vi "Steuerprogramm-01-17.vi"() -> ()   [LabVIEW 2010]
uses:
  <vilib>/rvi/interface/nirviReadWriteControl/nirviReadWriteControl.xnode
  <vilib>/rvi/errors/niLvFpgaWhatHappensToTopLevelVI.ctl
  <vilib>/rvi/interface/common/niFpgaNodeNameForErrorReporting.ctl
  <vilib>/rvi/errors/niLvFpgaAdjustHostInterfaceError.vi
  gvbooleschRT.vi
  <vilib>/rvi/interface/nirviCloseFPGA/nirviCloseFPGA.xnode
  GVMWHorst.vi
  GVMethodenwechsel.vi
  GVHorstSP.vi
  GVZwangs.vi
  GVHK1Hz.vi
  GVHeizenLH.vi
  GVAIs.vi
  GVTrapsMachs.vi
  GVaktuelleTDMS.vi
  GVECDs.vi
  GVZeitenZyklen.vi
  GVProbenvol.vi
  GVVentilposition.vi
  <vilib>/rvi/interface/nirviMethod/nirviMethod.xnode
  GVChroms.vi
  GVMetavariablen.vi
  GVZwangsMPV.vi
  NiFpgaLv.dll
  <vilib>/Utility/error.llb/Error Cluster From Error Code.vi
  C:/Users/HAGAR-IV/Desktop/Zeugs/markus/version feb 2012/FPGA Bitfiles/pertrasgcfpga2_FPGATarget_FPGA-Programm-01_A75D3647.lvbitx
  C:/Users/HAGAR-IV/Desktop/Zeugs/Johnny/pertrasgc fpga/FPGA-Programm-01-17.vi
  <vilib>/FPGAPlugInAG/cRIO-9114/niLvFpga_Close_cRIO-9114.vi
  Emil/HAGAR V - Licor/control/Licor-Sequences.ctl
  Emil/HAGAR V - Licor/control/Licor-Pump.ctl
  Emil/Licor-Steuerung/LicorLI7000/conventions/Licor-Source.ctl
  Emil/Licor-Steuerung/LicorLI7000/LicorLI7000.lvlib
  Emil/HAGAR V - Licor/control/Licor-Parameter.ctl
panel:
  in  "Methode speichern":bool
  out "ZyklusNummernGesamt":i32[](array[numeric])
  in  "veränderte Methode benutzen":bool
  in  "Methode verändern":bool
  out "ZyklusNummern":i32[](array[numeric])
  out "Big Ben, Methodenzeit, Zykluszeit0, Zykluszeit1, Zykluszeit2A, Zykluszeit2B":i32[](array[numeric])
  in  "global stop RT":bool
  in  "Methode":i32(ring) items=["Bedingsmethode", "Startmethode", "Meßmodus", "Shut-up-Methode", "Test", "HAG2 1/2", "Startmethode", "HAG2 1/2 Aufwärmen"]
  in  "Registerkarte":T1(tab)
  out "AIs1":dbl[](array[numeric])
  out "AIs1":string[](array[string])
  out "AIs2":string[](array[string])
  out "AIs3":string[](array[string])
  out "AIs2":dbl[](array[numeric])
  out "AIs3":dbl[](array[numeric])
  out "Metavariablen":string[](array[string])
  out "Metavariablen":dbl[](array[numeric])
  out "MWHorst":dbl[](array[numeric])
  out "HorstRegler":string[](array[string])
  out "Ventilposition":i32=1 min=1 max=6 step=1
  out "Housekeeping1":cluster{dbl[], dbl[]}(graph)
  in  "Zeitachse1":i32(ring)=1 items=["Zykluszeit [s] Mod0", "Zykluszeit [s] Mod1", "Zykluszeit [s] Mod2A", "Zykluszeit [s] Mod2B"]
  in  "dargestellte Größe 1":i32(ring)=1 items=["T1-Trap1", "T1-Trap2", "T1-StirlingKühlkopf", "T1-PreCol1", "T1-PreCol2", "T1-MainCol1a", "T1-MainCol1b", "T1-MainCol2a", "T1-MainCol2b", "T1-Bronkhorst1a", "T1-Bronkhorst1b", "T1-Bronkhorst2a", "T1-Bronkhorst2b", "T1-2Pos1B", "T1-Spare9", "T1-2Pos1A", "T1-Spare10", "T1-TurboPump", "T1-StirlingPlatine", "T1-Spare5", "T1-Spare6", "T1-Spare7", "T1-Spare8", "F1-MFM1", "F1-MFM0D [mL]", "P1-MethaneHP", "P1-MethaneLP", "P1-Vacuum", "TurboSpeed", "I1-MS-AC", "I1-Trap1", "I1-Trap2", "T2-ECD1a", "T2-ECD1b", "T2-ECD2a", "T2-ECD2b", "T2-Col1a", "T2-Col1b", "T2-Col2a", "T2-Col2b", "T2-Spare1", "T2-Spare2", "T2-Oven_a", "T2-Oven_b", "T2-Spare3", "T2-Spare4", "T2-Spare5", "F2-MFM0", "F2-MFM2A", "F2-MFM2B", "P2-N2O_HP", "P2-N2O_LP", "P2-CO2_HP", "P2-CO2_LP", "AI-Spare1", "FL-MFM1000mL", "AI-Spare3", "AI-Spare4", "StirlingAlarm", "StirlingEmerg.", "AI-Spare7", "AI-Spare8", "AI-Spare9", "FL-MFM30mL", "T0-DC/DC5", "I0-24V_M0", "I0-48V_M1", "I0-24V_M1", "I0-28V_M2", "T0-Spare3", "T0-Spare2", "T0-Spare4", "T0-DC/DC7", "I0-20V_Laptop", "I0-28V_M1", "I0-24V_M2", "I0-12V_Licor", "T0-Spare1", "T0-Drier", "T0-Spare5", "F0-MFM0A [L]", "TL-Licor_a", "P0-Span-HP", "P0-spare1", "P0-Stickstoff-LP", "P0-Helium-LP", "P0-Cal-HP", "P0-P9Tavco[bar]", "F0-MFM0B [L]", "TL-Licor_b", "P0-Span-LP", "P0-spare2", "P0-Stickstoff-HP", "P0-Helium-HP", "P0-Cal-LP", "F0-MFM3", "TemperaturTrap1[°C]", "TemperaturTrap2[°C]", "TemperaturPreMach1[°C]", "TemperaturPreMach2[°C]", "TemperaturMainMach1[°C]", "TemperaturMainMach2[°C]", "PrC0", "PrC0-Licor", "PrC1-Säule2", "PrC1-Säule1", "MFC1-Sample", "MFC1-Methan", "PrC1-BackFlush1", "PrC1-BackFlush2", "MFC2A", "MFC2B", "MFC2C", "PrC2A", "MFC2D", "MFC2E", "PrC2B"]
  out "Housekeeping2":cluster{dbl[], dbl[]}(graph)
  in  "Zeitachse2":i32(ring)=1 items=["Zykluszeit [s] Mod0", "Zykluszeit [s] Mod1", "Zykluszeit [s] Mod2A", "Zykluszeit [s] Mod2B"]
  in  "dargestellte Größe 2":i32(ring)=1 items=["T1-Trap1", "T1-Trap2", "T1-StirlingKühlkopf", "T1-PreCol1", "T1-PreCol2", "T1-MainCol1a", "T1-MainCol1b", "T1-MainCol2a", "T1-MainCol2b", "T1-Bronkhorst1a", "T1-Bronkhorst1b", "T1-Bronkhorst2a", "T1-Bronkhorst2b", "T1-2Pos1B", "T1-Spare9", "T1-2Pos1A", "T1-Spare10", "T1-TurboPump", "T1-StirlingPlatine", "T1-Spare5", "T1-Spare6", "T1-Spare7", "T1-Spare8", "F1-MFM1", "F1-MFM0D [mL]", "P1-MethaneHP", "P1-MethaneLP", "P1-Vacuum", "TurboSpeed", "I1-MS-AC", "I1-Trap1", "I1-Trap2", "T2-ECD1a", "T2-ECD1b", "T2-ECD2a", "T2-ECD2b", "T2-Col1a", "T2-Col1b", "T2-Col2a", "T2-Col2b", "T2-Spare1", "T2-Spare2", "T2-Oven_a", "T2-Oven_b", "T2-Spare3", "T2-Spare4", "T2-Spare5", "F2-MFM0", "F2-MFM2A", "F2-MFM2B", "P2-N2O_HP", "P2-N2O_LP", "P2-CO2_HP", "P2-CO2_LP", "AI-Spare1", "FL-MFM1000mL", "AI-Spare3", "AI-Spare4", "StirlingAlarm", "StirlingEmerg.", "AI-Spare7", "AI-Spare8", "AI-Spare9", "FL-MFM30mL", "T0-DC/DC5", "I0-24V_M0", "I0-48V_M1", "I0-24V_M1", "I0-28V_M2", "T0-Spare3", "T0-Spare2", "T0-Spare4", "T0-DC/DC7", "I0-20V_Laptop", "I0-28V_M1", "I0-24V_M2", "I0-12V_Licor", "T0-Spare1", "T0-Drier", "T0-Spare5", "F0-MFM0A [L]", "TL-Licor_a", "P0-Span-HP", "P0-spare1", "P0-Stickstoff-LP", "P0-Helium-LP", "P0-Cal-HP", "P0-P9Tavco[bar]", "F0-MFM0B [L]", "TL-Licor_b", "P0-Span-LP", "P0-spare2", "P0-Stickstoff-HP", "P0-Helium-HP", "P0-Cal-LP", "F0-MFM3", "TemperaturTrap1[°C]", "TemperaturTrap2[°C]", "TemperaturPreMach1[°C]", "TemperaturPreMach2[°C]", "TemperaturMainMach1[°C]", "TemperaturMainMach2[°C]", "PrC0", "PrC0-Licor", "PrC1-Säule2", "PrC1-Säule1", "MFC1-Sample", "MFC1-Methan", "PrC1-BackFlush1", "PrC1-BackFlush2", "MFC2A", "MFC2B", "MFC2C", "PrC2A", "MFC2D", "MFC2E", "PrC2B"]
  out "Detektor 2":cluster{dbl[], dbl[]}[](graph)
  in  "Detektor":i32(ring) items=["ECD1", "ECD2"]
  in  "HK1YMin":dbl
  in  "HK1YMax":dbl=100.0
  in  "HK2YMin":dbl
  in  "HK2YMax":dbl=100.0
  in  "DetYMin":dbl
  in  "DetYMax":dbl=100.0
  out "schnelleAnzeige":cluster{dbl[], dbl[]}(graph)
  in  "TafelWischen!":bool
  in  "dargestellte Größe 3":i32(ring)=1 items=["TemperaturTrap1[°C]", "TemperaturTrap2[°C]", "TemperaturPreMach1[°C]", "TemperaturPreMach2[°C]", "TemperaturMainMach1[°C]", "TemperaturMainMach2[°C]", "PrC0", "PrC0-Licor", "PrC1-Säule2", "PrC1-Säule1", "MFC1-Sample", "MFC1-Methan", "PrC1-BackFlush1", "PrC1-BackFlush2", "MFC2A", "MFC2B", "MFC2C", "PrC2A", "MFC2D", "MFC2E", "PrC2B"]
  in  "An/Aus":bool
  in  "manual control":T3={"sequence manual"=enum."WAIT", "sequence manual ?"=FALSE}
  out "Licor-output":string[](array[string])
  out "graph":cluster{"X":dbl[], "Y":dbl[]}(graph)
  in  "Licor-parameter out":T4={"CO2 ref"=392.0, "CO2 span"=402.0, "H2O ref"=0.0, "H2O span"=0.0, "Zi"=1.2, "Zt"=0.0, "Zm"=0.0, "S"=1.0, "Temp [C]"=50.0, "Pressure [hPa]"=135.0, "Licor-Sources"=["CO2A W", "CO2B W", "H2OA W", "H2OB W", "T C", "T V", "P kPa", "P V", "RH %", "CO2A um/m", "CO2B um/m", "H2OA mm/m", "H2OB mm/m"], "Licor-Pump"="Off", "Zeitstempel"=timestamp(0 s since 1904-01-01)} {"Pressure [hPa]" format="%.2g"; "Temp [C]" format="%.2f"; "CO2 ref" format="%.2f"; "CO2 span" format="%.2g"; "H2O ref" format="%.2g"; "H2O span" format="%.2g"}
  in  "ServosWarmHigh (us)KaltHigh(us)":T7={"Servo1WarmHigh(us)"=1000, "Servo1KaltHigh(us)"=1000, "Servo2WarmHigh(us)"=2030, "Servo2KaltHigh(us)"=2030}
  out "TDMSwriteECD":errorcluster
  out "AIsFIFOread":errorcluster
  out "MWTrapsMachs":errorcluster
  out "TDMSwriteHK":errorcluster
  out "TDMScloseHK":errorcluster
  out "TDMSopenHK":errorcluster
  out "TDMScloseECD2":errorcluster
  out "TDMSopenECD2":errorcluster
  out "TDMScloseECD1":errorcluster
  out "TDMSopenECD1":errorcluster
  out "FIFOwriteRS485":errorcluster
  out "SerielleKomm.":errorcluster
  out "LH":errorcluster
  out "Zyklus":errorcluster
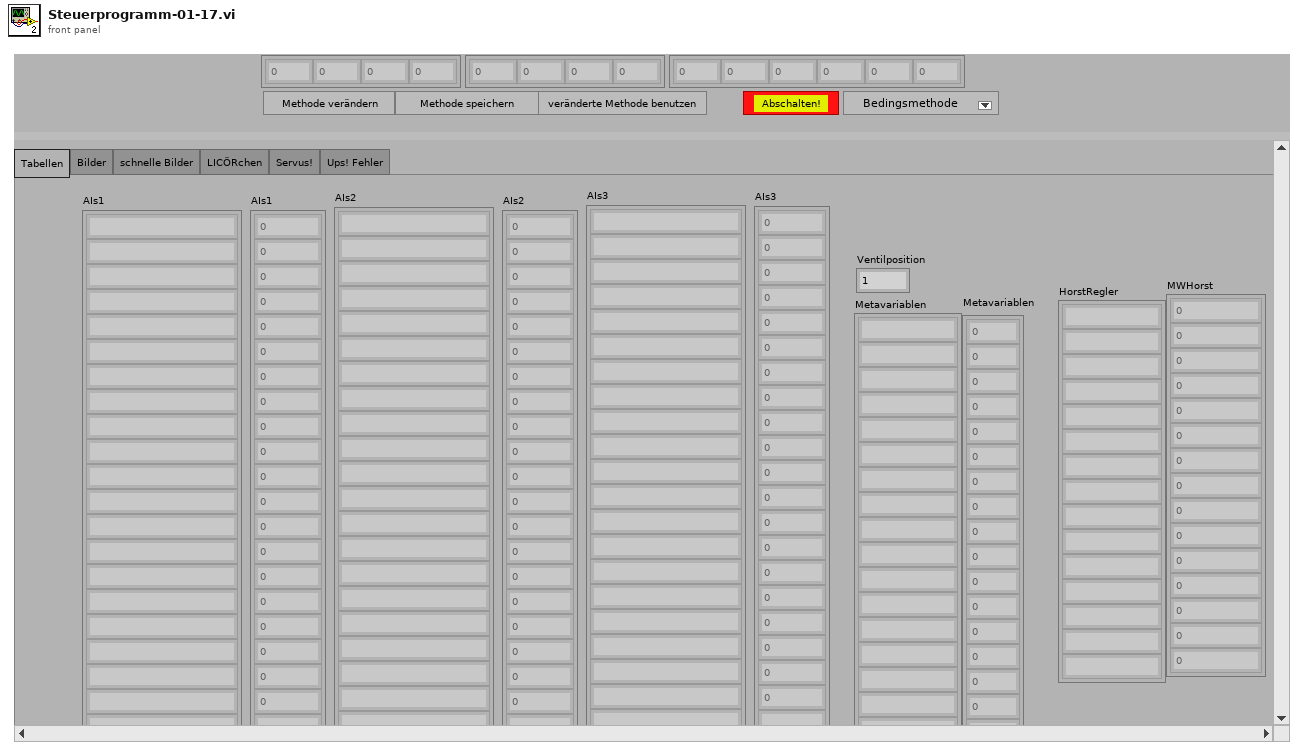
[diagram p1: front panel]
types:
  T1 = enum32{"Tabellen", "Bilder", "schnelle Bilder", "LICÖRchen", "Servus!", "Ups! Fehler"}
  T2 = typedef "Licor-Sequences.ctl" = enum16{"test", "WAIT", "warmup", "initialize", "calibrate Z", "calibrate S"}
  T3 = cluster{"sequence manual":T2, "sequence manual ?":bool}
  T4 = typedef "Licor-Parameter.ctl" = cluster{"CO2 ref":dbl, "CO2 span":dbl, "H2O ref":dbl, "H2O span":dbl, "Zi":dbl, "Zt":dbl, "Zm":dbl, "S":dbl, "Temp [C]":dbl, "Pressure [hPa]":dbl, "Licor-Sources":T5[], "Licor-Pump":T6, "Zeitstempel":timestamp}
  T5 = typedef "LicorLI7000.lvlib/Licor-Source.ctl" = string
  T6 = typedef "Licor-Pump.ctl" = string
  T7 = cluster{"Servo1WarmHigh(us)":u32, "Servo1KaltHigh(us)":u32, "Servo2WarmHigh(us)":u32, "Servo2KaltHigh(us)":u32}
  T8 = cluster{"DIOsMod0Nr":i32[], "DIOsMod1Nr":i32[], "DIOsMod2ANr":i32[], "DIOsMod2BNr":i32[], "AIsLH":i32[], "AnzahlRegler/Modul":i32[], "Regler für den Probenfluß":i32, "SPvorgebenMod0":string[], "SPvorgebenMod1":string[], "SPvorgebenMod2A":string[], "SPvorgebenMod2B":string[], "MWAntwortMod0":string[], "MWAntwortMod1":string[], "MWAntwortMod2A":string[], "MWAntwortMod2B":string[], "FaktorMod0":dbl[], "FaktorMod1":dbl[], "FaktorMod2A":dbl[], "FaktorMod2B":dbl[], "MWabfragenMod0":string[], "MWabfragenMod1":string[], "MWabfragenMod2A":string[], "MWabfragenMod2B":string[], "Modul1/AI koeff":dbl[][], "Modul2/AI koeff":dbl[][], "Modul3/AI koeff":dbl[][], "Traps/MachsKoeff":dbl[][], "Modul1/AIsNamen":string[], "Modul2/AIsNamen":string[], "Modul3/AIsNamen":string[], "DIOsMod0Name":string[], "DIOsMod1Name":string[], "DIOsMod2AName":string[], "DIOsMod2BName":string[], "ReglerNameMod0":string[], "ReglerNameMod1":string[], "ReglerNameMod2A":string[], "ReglerNameMod2B":string[], "Startmethode":i32, "Dateiordner Housekeeping":path, "Dateiname Housekeeping":string, "DateiordnerECD1":path, "DateinameECD1":string, "DateiordnerECD2":path, "DateinameECD2":string, "NamenLangsameHeizungen":string[], "ModuleLH":i32[], "Metavariablen":string[]}
  T9 = cluster{"Zykluslängen [s]":dbl[], "ZeitpktDIOsMod0":dbl[], "ZeitpktDIOsMod1":dbl[], "ZeitpktDIOsMod2A":dbl[], "ZeitpktDIOsMod2B":dbl[], "DIOsSPMod0":bool[][], "DIOsSPMod1":bool[][], "DIOsSPMod2A":bool[][], "DIOsSPMod2B":bool[][], "Mod0HorstZeitpkt":dbl[], "Mod1HorstZeitpkt":dbl[], "Mod2AHorstZeitpkt":dbl[], "Mod2BHorstZeitpkt":dbl[], "HorstSPMod0":dbl[][], "HorstSPMod1":dbl[][], "HorstSPMod2A":dbl[][], "HorstSPMod2B":dbl[][], "LHSetpoints":dbl[], "LHHeizen?":bool[], "ZPktFPGABoolesch":dbl[], "FPGABoolesch":bool[][], "ZeitpktFPGAPID":dbl[], "FPGAPID":cluster{"proportional gain (Kc)":fxp<+/-,16,8>, "integral gain (Kc*Ts/Ti)":fxp<+/-,16,8>, "derivative gain (Kc*Td/Ts)":fxp<+/-,16,8>}[][], "ZeitpktFPGAFixp":dbl[], "SHSetpoints":dbl[][], "t_PreMach1":dbl[], "T_PreMach1":dbl[], "t_PreMach2":dbl[], "T_PreMach2":dbl[], "PIDs für \"träge\" Heizungen":cluster{"proportional gain (Kc)":dbl, "integral time (Ti, min)":dbl, "derivative time (Td, min)":dbl}[], "Zwangsbedingungen":dbl[][], "Dateien fürs MS schicken?":bool, "ZeitpunkteMPV":dbl[], "SPMPV":i32[], "ZeitpktMS-1":dbl, "ZeitpktMS-2":dbl, "Int.Start1":dbl, "Int.Stop1":dbl, "Int.Start2":dbl, "Int.Stop2":dbl, "Methodenname":string, "t_MainMach1":dbl[], "T_MainMach1":dbl[], "t_MainMach2":dbl[], "T_MainMach2":dbl[]}[]
  T10 = enum16{"open", "replace", "create", "open or create", "replace or create", "replace or create with confirmation"}
  T11 = typedef "niFpgaNodeNameForErrorReporting.ctl" = enum16{"Open FPGA VI Reference", "Read/Write Control", "Invoke Method: Abort", "Invoke Method: Acknowledge IRQ", "Invoke Method: Download", "Invoke Method: FIFO.Configure", "Invoke Method: FIFO.Read", "Invoke Method: FIFO.Start", "Invoke Method: FIFO.Stop", "Invoke Method: FIFO.Write", "Invoke Method: Reset", "Invoke Method: Run", "Invoke Method: Wait on IRQ", "Close FPGA VI Reference"}
  T12 = typedef "niLvFpgaWhatHappensToTopLevelVI.ctl" = enum16{"top level VI scripted behind XNode", "top level VI inlined behind XNode"}
  T13 = cluster{"Zyklus1":i32, "Zeitachse1":i32, "dargestellte Größe 1":i32, "Zyklus2":i32, "Zeitachse2":i32, "dargestellte Größe 2":i32}
  T14 = cluster{"DIOsMod0Name":string[], "DIOsMod1Name":string[], "DIOsMod2AName":string[], "DIOsMod2BName":string[], "ReglerNameMod0":string[], "ReglerNameMod1":string[], "ReglerNameMod2A":string[], "ReglerNameMod2B":string[], "NamenLangsameHeizungen":string[]}
  T15 = cluster{"Zykluslängen [s]":dbl[], "ZeitpktDIOsMod0":dbl[], "ZeitpktDIOsMod1":dbl[], "ZeitpktDIOsMod2A":dbl[], "ZeitpktDIOsMod2B":dbl[], "DIOsSPMod0":bool[][], "DIOsSPMod1":bool[][], "DIOsSPMod2A":bool[][], "DIOsSPMod2B":bool[][], "Mod0HorstZeitpkt":dbl[], "Mod1HorstZeitpkt":dbl[], "Mod2AHorstZeitpkt":dbl[], "Mod2BHorstZeitpkt":dbl[], "HorstSPMod0":dbl[][], "HorstSPMod1":dbl[][], "HorstSPMod2A":dbl[][], "HorstSPMod2B":dbl[][], "LHSetpoints":dbl[], "LHHeizen?":bool[], "ZPktFPGABoolesch":dbl[], "FPGABoolesch":bool[][], "ZeitpktFPGAPID":dbl[], "FPGAPID":cluster{"proportional gain (Kc)":fxp<+/-,16,8>, "integral gain (Kc*Ts/Ti)":fxp<+/-,16,8>, "derivative gain (Kc*Td/Ts)":fxp<+/-,16,8>}[][], "ZeitpktFPGAFixp":dbl[], "SHSetpoints":dbl[][], "t_PreMach1":dbl[], "T_PreMach1":dbl[], "t_PreMach2":dbl[], "T_PreMach2":dbl[], "PIDs für \"träge\" Heizungen":cluster{"proportional gain (Kc)":dbl, "integral time (Ti, min)":dbl, "derivative time (Td, min)":dbl}[], "Zwangsbedingungen":dbl[][], "Dateien fürs MS schicken?":bool, "ZeitpunkteMPV":dbl[], "SPMPV":i32[], "ZeitpktMS-1":dbl, "ZeitpktMS-2":dbl, "Int.Start1":dbl, "Int.Stop1":dbl, "Int.Start2":dbl, "Int.Stop2":dbl, "Methodenname":string, "t_MainMach1":dbl[], "T_MainMach1":dbl[], "t_MainMach2":dbl[], "T_MainMach2":dbl[]}
  T16 = cluster{"created path":path, "created path":path, "created path":path, "Dateiname Housekeeping":string, "DateinameECD1":string, "DateinameECD2":string, "tdms0":refnum<k34>, "tdms1":refnum<k34>, "tdms0":refnum<k34>, "tdms1":refnum<k34>, "tdms0":refnum<k34>, "tdms1":refnum<k34>}
  T17 = cluster{"proportional gain (Kc)":fxp<+/-,16,8>, "integral gain (Kc*Ts/Ti)":fxp<+/-,16,8>, "derivative gain (Kc*Td/Ts)":fxp<+/-,16,8>}[][]
  T18 = cluster{"proportional gain (Kc)":dbl, "integral time (Ti, min)":dbl, "derivative time (Td, min)":dbl}[]
  T19 = cluster{cluster{"ZeitpktDIOsMod2B":dbl[]}[], cluster{"DIOsSPMod2B":bool[][]}[], cluster{"Mod2BHorstZeitpkt":dbl[]}[], cluster{"HorstSPMod2B":dbl[][]}[], "LHHeizen?":bool[], "ZPktFPGABoolesch":dbl[], "FPGABoolesch":bool[][], "ZeitpktFPGAPID":dbl[], "FPGAPID":cluster{"proportional gain (Kc)":fxp<+/-,16,8>, "integral gain (Kc*Ts/Ti)":fxp<+/-,16,8>, "derivative gain (Kc*Td/Ts)":fxp<+/-,16,8>}[][], "ZeitpktFPGAFixp":dbl[], "SHSetpoints":dbl[][], "t_PreMach1":dbl[], "T_PreMach1":dbl[], "t_PreMach2":dbl[], "T_PreMach2":dbl[], "ZeitpunkteMPV":dbl[], "SPMPV":i32[], "t_MainMach1":dbl[], "T_MainMach1":dbl[], "t_MainMach2":dbl[], "T_MainMach2":dbl[]}
  T20 = cluster{"Zykluslängen [s]":dbl[], "ZeitpktDIOsMod0":dbl[], "ZeitpktDIOsMod1":dbl[], "ZeitpktDIOsMod2A":dbl[], "ZeitpktDIOsMod2B":dbl[], "DIOsSPMod0":bool[][], "DIOsSPMod1":bool[][], "DIOsSPMod2A":bool[][], "DIOsSPMod2B":bool[][], "Mod0HorstZeitpkt":dbl[], "Mod1HorstZeitpkt":dbl[], "Mod2AHorstZeitpkt":dbl[], "Mod2BHorstZeitpkt":dbl[], "HorstSPMod0":dbl[][], "HorstSPMod1":dbl[][], "HorstSPMod2A":dbl[][], "HorstSPMod2B":dbl[][], "LangsameHeizungenSP":dbl[], "LHHeizen?":bool[], "ZPktFPGABoolesch":dbl[], "FPGABoolesch":bool[][], "ZeitpktFPGAPID":dbl[], "FPGAPID":cluster{"proportional gain (Kc)":fxp<+/-,16,8>, "integral gain (Kc*Ts/Ti)":fxp<+/-,16,8>, "derivative gain (Kc*Td/Ts)":fxp<+/-,16,8>}[][], "ZeitpktFPGAFixp":dbl[], "FPGAFixp":dbl[][], "t_PreMach1":dbl[], "T_PreMach1":dbl[], "t_PreMach2":dbl[], "T_PreMach2":dbl[], "PIDs für \"träge\" Heizungen":cluster{"proportional gain (Kc)":dbl, "integral time (Ti, min)":dbl, "derivative time (Td, min)":dbl}[], "Zwangsbedingungen":dbl[][], "MS-Daten?":bool, "ZeitpunkteMPV":dbl[], "SetpointMPV":i32[], "ZeitpktMS-1":dbl, "ZeitpktMS-2":dbl, "Int.Start1":dbl, "Int.Stop1":dbl, "Int.Start2":dbl, "Int.Stop2":dbl, "Methodenname":string, "t_MainMach1":dbl[], "T_MainMach1":dbl[], "t_MainMach2":dbl[], "T_MainMach2":dbl[]}
  T21 = cluster{"ZyklusNummern":i32[], "ZeilennummernDIOs":i32[], "ZwangsDIO?":cluster{bool[]}[], "ZeilennummernHorst":i32[], "ZwangsHorst?":cluster{bool[]}[], "ZeileFPGABoolesch":i32, "ZwangsFPGABoolesch?":bool[], "ZeileFPGAPID":i32, "ZeileFPGAFixp":i32, "ZeilePreMach1":i32, "ZeilePreMach2":i32, "ZeilennummerMPV":i32, "ZeileMainMach1":i32, "ZeileMainMach2":i32, "ZwangsMPV?":bool}
  T22 = cluster{"ZyklusNummern":i32[], i32[], "ZwangsDIO?":cluster{bool[]}[], i32[], "ZwangsHorst?":cluster{bool[]}[], i32, "ZwangsFPGABoolesch?":bool[], i32, i32, "ZeileMach":i32, "ZeileMach":i32, i32, "ZeileMach":i32, "ZeileMach":i32, "ZwangsMPV?":bool}
  T23 = cluster{string[], string[], string[], dbl[], dbl[], dbl[]}
  T24 = cluster{"Befehle1":string[], "Befehle2":string[], "Befehle3":string[]}
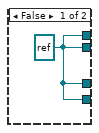
[diagram p2: hidden frame]
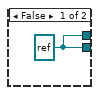
[diagram p3: hidden frame]
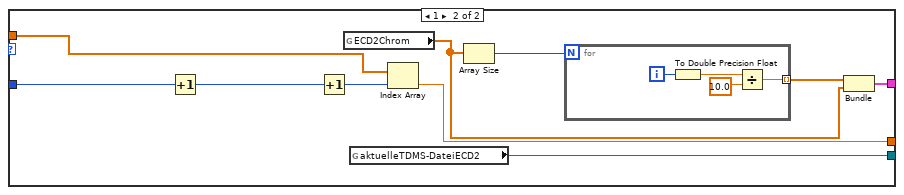
[diagram p13: hidden frame]
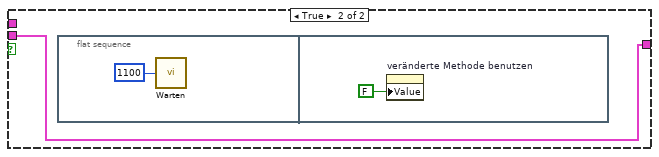
[diagram p14: hidden frame]
diagram:
  n1 = Open/Create/Replace File(file path (use dialog)=path "c:/einstellungen.per" ("Datei (Dialog verwenden)"), operation (0:open)=T10."open" ("Operation (0:Öffnen)")) -> (refnum out=w12:refnum<file>)  [unwired: 4 in, 2 out]
  n2 = Open/Create/Replace File(file path (use dialog)=path "c:/methoden.per" ("Datei (Dialog verwenden)"), operation (0:open)=T10."open" ("Operation (0:Öffnen)")) -> (refnum out=w7:refnum<file>)  [unwired: 4 in, 2 out]
  n3 = Read from Binary File(5:T8 {"DIOsMod0Nr"=[], "DIOsMod1Nr"=[], "DIOsMod2ANr"=[], "DIOsMod2BNr"=[], "AIsLH"=[], "AnzahlRegler/Modul"=[], "Regler für den Probenfluß"=0, "SPvorgebenMod0"=[], "SPvorgebenMod1"=[], "SPvorgebenMod2A"=[], "SPvorgebenMod2B"=[], "MWAntwortMod0"=[], "MWAntwortMod1"=[], "MWAntwortMod2A"=[], "MWAntwortMod2B"=[], "FaktorMod0"=[], "FaktorMod1"=[], "FaktorMod2A"=[], "FaktorMod2B"=[], "MWabfragenMod0"=[], "MWabfragenMod1"=[], "MWabfragenMod2A"=[], "MWabfragenMod2B"=[], "Modul1/AI koeff"=[], "Modul2/AI koeff"=[], "Modul3/AI koeff"=[], "Traps/MachsKoeff"=[], "Modul1/AIsNamen"=[], "Modul2/AIsNamen"=[], "Modul3/AIsNamen"=[], "DIOsMod0Name"=[], "DIOsMod1Name"=[], "DIOsMod2AName"=[], "DIOsMod2BName"=[], "ReglerNameMod0"=[], "ReglerNameMod1"=[], "ReglerNameMod2A"=[], "ReglerNameMod2B"=[], "Startmethode"=0, "Dateiordner Housekeeping"=path "", "Dateiname Housekeeping"="", "DateiordnerECD1"=path "", "DateinameECD1"="", "DateiordnerECD2"=path "", "DateinameECD2"="", "NamenLangsameHeizungen"=[], "ModuleLH"=[], "Metavariablen"=[]} ("Ausgangs-Cluster"), 11:w12) -> (2:w10:T8, 3:w11:refnum<file>)  [unwired: 4 in, 2 out]
  n4 = Read from Binary File(5:T9 [], 11:w7) -> (2:w5:T9, 3:w6:refnum<file>)  [unwired: 4 in, 2 out]
  n5 = Close File(refnum=w11) -> ()  [unwired: 1 in, 2 out]
  n6 = Close File(refnum=w6) -> ()  [unwired: 1 in, 2 out]
  n7 = flat-sequence {
    tunnel: [w41] -> w40
    tunnel: [w98] -> w39
    tunnel: [w45] -> w37
    tunnel: [w232] -> w36
    tunnel: [w234] -> w35
    tunnel: [w226] -> w34
    tunnel: [w233] -> w33
    tunnel: [w156] -> w32
    tunnel: [w225] -> w31
    tunnel: [w224] -> w30
    tunnel: [w218] -> w29
    tunnel: [w159] -> w28
    tunnel: [w133] -> w27
    tunnel: [w231] -> w26
    tunnel: [w223] -> w25
    tunnel: [w222] -> w24
    tunnel: [w214] -> w23
    tunnel: [w213] -> w22
    tunnel: [w212] -> w21
    tunnel: [w211] -> w20
    tunnel: [w210] -> w19
    tunnel: [w209] -> w18
    tunnel: [w206] -> w17
    tunnel: [w188] -> w16
    tunnel: w10 -> [w74]
    tunnel: [w187] -> w15
    tunnel: w5 -> [w99]
    tunnel: [w98] -> w4
    tunnel: [w74] -> w1
    tunnel: w40 -> [w430]
    tunnel: w39 -> [w503]
    tunnel: [w430] -> w38
    tunnel: w37 -> [_]
    tunnel: w36 -> [w461]
    tunnel: w35 -> [w460]
    tunnel: w34 -> [w462]
    tunnel: w33 -> [w459]
    tunnel: w32 -> [w434]
    tunnel: w31 -> [w429]
    tunnel: w30 -> [w426]
    tunnel: w29 -> [w423]
    tunnel: w28 -> [w424]
    tunnel: w27 -> [w427]
    tunnel: w26 -> [w501]
    tunnel: w25 -> [w432]
    tunnel: w24 -> [w502]
    tunnel: w23 -> [w405]
    tunnel: w22 -> [w404]
    tunnel: w21 -> [w403]
    tunnel: w20 -> [w499]
    tunnel: w19 -> [w498]
    tunnel: w18 -> [w497]
    tunnel: w17 -> [w451]
    tunnel: w16 -> [w433]
    tunnel: w15 -> [w422]
    tunnel: w5 -> [w421]
    tunnel: w4 -> [w419]
    tunnel: w1 -> [_]
    tunnel: w38 -> [w1270]
    frame #0 {
      w100 = TRUE
      w115 = 0.0 ("Probenvol.1")
      w122 = dbl[] [-1.0] ("ECD1MW")
      w123 = FALSE ("ECD1Empfangen?")
      w114 = string[] ["TemperaturTrap1[°C]", "TemperaturTrap2[°C]", "TemperaturPreMach1[°C]", "TemperaturPreMach2[°C]", "TemperaturMainMach1[°C]", "TemperaturMainMach2[°C]"]
      w229 = string[] ["Big Ben [s]", "Methodenzeit [s]", "Zykluszeit [s] Mod0", "Zykluszeit [s] Mod1", "Zykluszeit [s] Mod2A", "Zykluszeit [s] Mod2B"]
      w219 = FALSE ("Undefinierte Werte möglich")
      w220 = FALSE ("global stop RT")
      n8 = for {
        tunnel: [w394] -> w227 mode=indexing
        tunnel: w99 -> [w395] mode=indexing
        n9 = Unbundle(w395) -> ("Methodenname"=w394:string)  [unwired: 44 out]
      }
      n10 = call "FPGA-Start-01-17.vi"() -> ("error out"=w45:errorcluster, "FPGA VI Reference Out"=w44:refnum<k20>)  [unwired: 2 in]
      n11 = Unbundle(w74) -> ("DIOsMod0Nr"=w143:i32[], "DIOsMod1Nr"=w142:i32[], "DIOsMod2ANr"=w141:i32[], "DIOsMod2BNr"=w140:i32[], "AIsLH"=w130:i32[], "AnzahlRegler/Modul"=w133:i32[], "Regler für den Probenfluß"=w187:i32, "SPvorgebenMod0"=w186:string[], "SPvorgebenMod1"=w185:string[], "SPvorgebenMod2A"=w184:string[], "SPvorgebenMod2B"=w183:string[], "MWAntwortMod0"=w182:string[], "MWAntwortMod1"=w181:string[], "MWAntwortMod2A"=w180:string[], "MWAntwortMod2B"=w179:string[], "FaktorMod0"=w178:dbl[], "FaktorMod1"=w177:dbl[], "FaktorMod2A"=w176:dbl[], "FaktorMod2B"=w175:dbl[], "MWabfragenMod0"=w174:string[], "MWabfragenMod1"=w173:string[], "MWabfragenMod2A"=w172:string[], "MWabfragenMod2B"=w171:string[], "Modul1/AI koeff"=w170:dbl[][], "Modul2/AI koeff"=w169:dbl[][], "Modul3/AI koeff"=w168:dbl[][], "Traps/MachsKoeff"=w167:dbl[][], "Modul1/AIsNamen"=w166:string[], "Modul2/AIsNamen"=w165:string[], "Modul3/AIsNamen"=w164:string[], "DIOsMod0Name"=w72:string[], "DIOsMod1Name"=w73:string[], "DIOsMod2AName"=w71:string[], "DIOsMod2BName"=w70:string[], "ReglerNameMod0"=w89:string[], "ReglerNameMod1"=w88:string[], "ReglerNameMod2A"=w87:string[], "ReglerNameMod2B"=w86:string[], "Startmethode"=w98:i32, "Dateiordner Housekeeping"=w69:path, "Dateiname Housekeeping"=w163:string, "DateiordnerECD1"=w83:path, "DateinameECD1"=w162:string, "DateiordnerECD2"=w82:path, "DateinameECD2"=w161:string, "NamenLangsameHeizungen"=w160:string[], "ModuleLH"=w155:i32[], "Metavariablen"=w93:string[])
      "Metavariablen" <- w93
      n12 = Initialize Array(0, 4 ("Dimension")) -> (w116:i32[])
      n13 = Initialize Array(0.0 ("Element"), 6 ("Dimension")) -> (w119:dbl[])
      n14 = global write "GVMethodenwechsel.vi" "Methodenwechsel?"(FALSE ("Methodenwechsel?")) -> ()
      n15 = Concatenate Strings("?SE0,SETP,2200" ("string"), "\r\n") -> (w47:string)
      n16 = Concatenate Strings("?SE0,SETP,2300" ("string"), "\r\n") -> (w54:string)
      n17 = String To Byte Array(string=w54) -> (unsigned byte array=w59:u8[])
      n18 = Join Numbers(hi=w59, lo=u8 6) -> ((hi.lo)=w57:u16[])
      n19 = String To Byte Array(string=w47) -> (unsigned byte array=w49:u8[])
      n20 = Join Numbers(hi=w49, lo=u8 5) -> ((hi.lo)=w46:u16[])
      n21 = xnode "Invoke Method"("FPGA VI Reference In"=w44, "Data"=w46) -> ("FPGA VI Reference Out"=w52:refnum<k20>)  [unwired: 2 in, 2 out]
      n22 = xnode "Invoke Method"("FPGA VI Reference In"=w52, "Data"=w57) -> ("FPGA VI Reference Out"=w43:refnum<k20>)  [unwired: 2 in, 2 out]
      n23 = global write "GVProbenvol.vi" "Probenvol.1"(w115) -> ()
      n24 = global write "GVProbenvol.vi" "Probenvol.2"(w115) -> ()
      n25 = global write "GVECDs.vi" "ECD1MW"(w122) -> ()
      n26 = global write "GVECDs.vi" "ECD2MW"(w122) -> ()
      n27 = global write "GVECDs.vi" "ECD1Empfangen?"(w123) -> ()
      n28 = global write "GVECDs.vi" "ECD2Empfangen?"(w123) -> ()
      n29 = property on="dargestellte Größe 2" class="Ring (strict)"("AllowUndefVals"=w219) -> ()  [unwired: 2 in, 2 out]
      n30 = property on="Zeitachse2" class="Ring (strict)"("AllowUndefVals"=w219) -> ()  [unwired: 2 in, 2 out]
      n31 = property on="Zeitachse1" class="Ring (strict)"("AllowUndefVals"=w219) -> ()  [unwired: 2 in, 2 out]
      n32 = property on="dargestellte Größe 1" class="Ring (strict)"("AllowUndefVals"=w219) -> ()  [unwired: 2 in, 2 out]
      n33 = property on="Methode" class="Ring (strict)"("AllowUndefVals"=w219) -> ()  [unwired: 2 in, 2 out]
      n34 = local write "global stop RT"(w220) -> ()
      n35 = global write "gvbooleschRT.vi" "global stop RT"(w220) -> ()
      n36 = global write "GVZeitenZyklen.vi" "ZyklusNummern"(w116) -> ()
      n37 = global write "GVZeitenZyklen.vi" "ZyklusNummernGesamt"(w116) -> ()
      n38 = global write "GVZeitenZyklen.vi" "Big Ben, Methodenzeit, Zykluszeit0, Zykluszeit1, Zykluszeit2A, Zykluszeit2B"(w119) -> ()
      n39 = property on="Methode" class="Ring (strict)"("Value"=w98) -> ()  [unwired: 2 in, 2 out]
      n40 = call "MPVSenden-01-17.vi"("Ventilposition"=0, "FPGA VI Reference In"=w43) -> ("FPGA VI Reference Out"=w41:refnum<k20>)  [unwired: 1 in, 2 out]
      n41 = Initialize Array(-1.0 ("Element"), 6 ("Dimension")) -> (w126:dbl[])
      n42 = Initialize Array(FALSE, 10 ("Dimension")) -> (w134:bool[])
      n43 = Initialize Array(-1.0 ("Element"), 96 ("Dimension")) -> (w127:dbl[])
      n44 = global write "GVZwangs.vi" "ZwangsFPGABoolesch!"(w134) -> ()
      n45 = global write "GVZwangs.vi" "ZwangsFPGABoolesch?"(w134) -> ()
      n46 = global write "GVTrapsMachs.vi" "Traps/Machs"(w126) -> ()
      n47 = global write "GVAIs.vi" "AIs"(w127) -> ()
      n48 = for {
        tunnel: w133 -> [w372] mode=indexing
        tunnel: [w369] -> w132 mode=indexing
        tunnel: [w367] -> w131 mode=indexing
        n49 = Initialize Array(0.0 ("Element"), w372) -> (w370:dbl[])
        n50 = Initialize Array(FALSE, w372) -> (w368:bool[])
        n51 = Bundle(w370) -> (w369:cluster{dbl[]})  [unwired: 1 in]
        n52 = Bundle(w368) -> (w367:cluster{bool[]})  [unwired: 1 in]
      }
      n53 = Bundle("DIOsMod0Name"=w72, "DIOsMod1Name"=w73, "DIOsMod2AName"=w71, "DIOsMod2BName"=w70, "ReglerNameMod0"=w89, "ReglerNameMod1"=w88, "ReglerNameMod2A"=w87, "ReglerNameMod2B"=w86, "NamenLangsameHeizungen"=w160) -> (w222:T14)  [unwired: 1 in]
      n54 = Build Array (concatenate)(w89, w88, w87, w86) -> (w113:string[])
      n55 = Build Array (concatenate)(w182, w181, w180, w179) -> (w233:string[])
      n56 = Build Array (concatenate)(w186, w185, w184, w183) -> (w234:string[])
      n57 = Build Array (concatenate)(w178, w177, w176, w175) -> (w226:dbl[])
      n58 = Build Array (concatenate)(w174, w173, w172, w171) -> (w232:string[])
      n59 = Build Array (concatenate)(w89, w88, w87, w86) -> (→"HorstRegler":string[])
      n60 = Array Size(array=w93) -> (size(s)=w92:i32)
      n61 = Build Array(w143, w142, w141, w140) -> (w139:i32[][])
      n62 = Array Size(array=w160) -> (size(s)=w159:i32)
      n63 = Add Array Elements(numeric array=w133) -> (sum=w218:i32)
      n64 = Array Size(array=w130) -> (size(s)=w129:i32)
      n65 = Index Array(array=w99, index=w98) -> (element=w97:T15)
      n66 = Add Array Elements(numeric array=w133) -> (sum=w145:i32)
      n67 = Build Cluster Array(w143, w142, w141, w140) -> (w225:cluster{"DIOsMod2BNr":i32[]}[])
      n68 = Decrement(x=w155) -> (x-1=w154:i32[])
      n69 = Build Array (concatenate)(w166, w165, w164) -> (w104:string[])
      n70 = Index Array(array=w167, index (col)=0 ("Deaktivierter Index (Spalte)")) -> (element=w212:dbl[])  [unwired: 1 in]
      n71 = Index Array(array=w167, index (col)=1 ("Deaktivierter Index (Spalte)")) -> (element=w213:dbl[])  [unwired: 1 in]
      n72 = Index Array(array=w167, index (col)=2 ("Deaktivierter Index (Spalte)")) -> (element=w214:dbl[])  [unwired: 1 in]
      n73 = for {
        tunnel: w225 -> [w397] mode=indexing
        tunnel: [w398] -> w224 mode=indexing
        n74 = Unbundle(w397) -> ("DIOsMod2BNr"=w396:i32[])
        n75 = Array Size(array=w396) -> (size(s)=w398:i32)
      }
      n76 = property on="Methode" class="Ring (strict)"("Strings []"=w227) -> ()  [unwired: 2 in, 2 out]
      n77 = Build Array (concatenate)(w127, w126) -> (w125:dbl[])
      n78 = Array Size(array=w139) -> (size(s)=w138:i32[])
      n79 = Unbundle(w97) -> ("SPMPV"=w96:i32[])  [unwired: 44 out]
      n80 = Open/Create/Replace File(file path (use dialog)=path "c:/fromcriordy.txt" ("Dateipfad (Dialog verwenden)"), operation (0:open)=T10."replace or create" ("Operation (0:Öffnen)")) -> (refnum out=w191:refnum<file>, error out=w192:errorcluster)  [unwired: 4 in, 1 out]
      n81 = Initialize Array(0.0 ("Element"), w145) -> (w144:dbl[])
      n82 = Initialize Array(0.0 ("element"), w92) -> (w90:dbl[])
      n83 = Get Date/Time In Seconds() -> (seconds since 1Jan1904=w84:timestamp)
      n84 = Initialize Array(FALSE, w129) -> (w124:bool[])
      n85 = Multiply(x=w154, y=32) -> (x*y=w157:i32[])
      n86 = Initialize Array(-1.0, w145) -> (w147:dbl[])
      n87 = Array Subset(array=w104, index=32 ("Index"), length=32 ("Länge")) -> (→"AIs2":string[])
      n88 = Array Subset(array=w104, index=0 ("Index"), length=32 ("Länge")) -> (→"AIs1":string[])
      n89 = Array Subset(array=w104, index=64 ("Index"), length=32 ("Länge")) -> (→"AIs3":string[])
      n90 = global write "GVHK1Hz.vi" "Mod1Mod2Mod3/AITrapsMachs1Hz"(w125) -> ()
      n91 = global write "GVHorstSP.vi" "HorstSP"(w144) -> ()
      n92 = for {
        tunnel: w138 -> [w377] mode=indexing
        tunnel: [w374] -> w137 mode=indexing
        n93 = Initialize Array(FALSE, w377) -> (w375:bool[])
        n94 = Bundle(w375) -> (w374:cluster{bool[]})  [unwired: 1 in]
      }
      n95 = global write "GVMetavariablen.vi" "Metavariablen"(w90) -> ()
      n96 = global write "GVHeizenLH.vi" "Heizen?LH"(w124) -> ()
      n97 = global write "GVZwangs.vi" "ZwangsLangsameH!"(w124) -> ()
      n98 = global write "GVZwangs.vi" "ZwangsLangsameH?"(w124) -> ()
      n99 = Add(x=w157, y=w130) -> (x+y=w156:i32[])
      n100 = Close File(refnum=w191, error in=w192) -> (path=w223:path)  [unwired: 1 out]
      n101 = Format Date/Time String(time format string (%c)="%Y-%m-%d--%H-%M" ("Zeitformatierungs-String (%c)"), seconds (now)=w84) -> (date/time string=w62:string)  [unwired: 1 in]
      n102 = Index Array(array=w96, index=0) -> (element=w94:i32)
      n103 = global write "GVMWHorst.vi" "MWHorst"(w147) -> ()
      n104 = global write "GVVentilposition.vi" "Ventilposition"(w94) -> ()
      n105 = Build Array (concatenate)(string[] ["Jahr", "Monat", "Tag", "Stunde", "Minute", "Sekunde"] ("Array"), string[] ["Datei Nr.", "Methode Nr.", "Zyklusnr. Mod0", "Zyklusnr. Mod1", "Zyklusnr. Mod2A", "Zyklusnr. Mod2B"], w229, w104, w114, w113, "Probenvolumen1", "Probenvolumen2", "Ventilposition" ("element"), string[] ["CPU Total", "CPU Time critical", "CPU Timed Structures", "CPU High", "CPU Above normal", "CPU Normal", "CPU Background", "CPU Idle", "CPU ISR", "Memory", "SekundenTotalBrutal"]) -> (w231:string[])
      n106 = Build Array (concatenate)(w114, w113) -> (w112:string[])
      n107 = Build Array (concatenate)(w104, w114, w113) -> (w111:string[])
      n108 = Split 1D Array(array=w229, index=2 ("Index")) -> (second subarray=w221:string[])  [unwired: 1 out]
      n109 = Concatenate Strings("HK " ("String"), w62) -> (w66:string)
      n110 = Concatenate Strings("ECD1 " ("String"), w62) -> (w64:string)
      n111 = Concatenate Strings("ECD2 " ("String"), w62) -> (w61:string)
      n112 = property on="dargestellte Größe 1" class="Ring (strict)"("Strings []"=w111) -> ()  [unwired: 2 in, 2 out]
      n113 = property on="Zeitachse2" class="Ring (strict)"("Strings []"=w221) -> ()  [unwired: 2 in, 2 out]
      n114 = property on="Zeitachse1" class="Ring (strict)"("Strings []"=w221) -> ()  [unwired: 2 in, 2 out]
      n115 = property on="dargestellte Größe 3" class="Ring (strict)"("Strings []"=w112) -> ()  [unwired: 2 in, 2 out]
      n116 = global write "GVZwangs.vi" "ZwangsHorst!"(w132) -> ()
      n117 = property on="dargestellte Größe 2" class="Ring (strict)"("Strings []"=w111) -> ()  [unwired: 2 in, 2 out]
      n118 = global write "GVZwangs.vi" "ZwangsHorst?"(w131) -> ()
      n119 = Build Path(base path=w69, name or relative path=w66) -> (appended path=w77:path)
      n120 = Build Path(base path=w83, name or relative path=w64) -> (appended path=w79:path)
      n121 = Build Path(base path=w82, name or relative path=w61) -> (appended path=w81:path)
      n122 = Create Folder(path (use dialog)=w77) -> (created path=w76:path)  [unwired: 2 in, 2 out]
      n123 = Create Folder(path (use dialog)=w79) -> (created path=w78:path)  [unwired: 2 in, 2 out]
      n124 = Create Folder(path (use dialog)=w81) -> (created path=w80:path)  [unwired: 2 in, 2 out]
      n125 = global write "GVZwangs.vi" "ZwangsDIO!"(w137) -> ()
      n126 = global write "GVZwangs.vi" "ZwangsDIO?"(w137) -> ()
      n127 = case shown="True" w100 {
        tunnel: [w388 w393] -> w205
        tunnel: [w388 w392] -> w204
        tunnel: w76 -> [_ w391]
        tunnel: w163 -> [_ w390]
        tunnel: w98 -> [_ w389]
        frame False {
          w388 = refnum<k34> refnum ("tdms1")
        }
        frame True {
          n128 = call "TDMS0.vi"("Startmethode"=w389, "Dateiname"=w390, "Dateiordner"=w391) -> ("tdms1"=w392:refnum<k34>, "tdms0"=w393:refnum<k34>)
          n129 = global write "GVaktuelleTDMS.vi" "aktuelleTDMS-DateiHK"(w393) -> ()
        }
      }
      n130 = case shown="True" w100 {
        tunnel: [w378 w387] -> w203
        tunnel: [w378 w386] -> w202
        tunnel: [w378 w385] -> w201
        tunnel: [w378 w384] -> w200
        tunnel: w78 -> [_ w383]
        tunnel: w162 -> [_ w382]
        tunnel: w80 -> [_ w381]
        tunnel: w161 -> [_ w380]
        tunnel: w98 -> [_ w379]
        frame False {
          w378 = refnum<k34> refnum ("tdms0")
        }
        frame True {
          n131 = call "TDMS0.vi"("Startmethode"=w379, "Dateiname"=w382, "Dateiordner"=w383) -> ("tdms1"=w386:refnum<k34>, "tdms0"=w387:refnum<k34>)
          n132 = call "TDMS0.vi"("Startmethode"=w379, "Dateiname"=w380, "Dateiordner"=w381) -> ("tdms1"=w384:refnum<k34>, "tdms0"=w385:refnum<k34>)
          n133 = global write "GVaktuelleTDMS.vi" "aktuelleTDMS-DateiECD1"(w387) -> ()
          n134 = global write "GVaktuelleTDMS.vi" "aktuelleTDMS-DateiECD2"(w385) -> ()
        }
      }
      n135 = Open/Create/Replace File(file path (use dialog)=path "c:/fromcriocmd.txt" ("Pfad MS-Datei CRIO"), operation (0:open)=T10."replace or create" ("Operation (0:Öffnen)")) -> (refnum out=w197:refnum<file>, error out=w196:errorcluster)  [unwired: 4 in, 1 out]
      n136 = call "AIKoeffSortieren.vi"("Modul3/AI koeff"=w168, "Modul2/AI koeff"=w169, "Modul1/AI koeff"=w170) -> ("P0"=w209:dbl[], "P1"=w210:dbl[], "P2"=w211:dbl[])
      n137 = Write to Text File(file (use dialog)=w197, text="time=yyyymmddhhmmss\ncycle=005\ninfo=1234567890123456789012345678901234567890123456789012345678901234567890123456789012345678901234567890\nlength=100\ncmd=cycle" ("Text0 MS-Datei"), error in=w196) -> (refnum out=w194:refnum<file>, error out=w193:errorcluster)  [unwired: 1 in, 1 out]
      n138 = Bundle("created path"=w76, "created path"=w78, "created path"=w80, "Dateiname Housekeeping"=w163, "DateinameECD1"=w162, "DateinameECD2"=w161, "tdms0"=w205, "tdms1"=w204, "tdms0"=w203, "tdms1"=w202, "tdms0"=w201, "tdms1"=w200) -> (w206:T16)  [unwired: 1 in]
      n139 = Close File(refnum=w194, error in=w193) -> (path=w188:path)  [unwired: 1 out]
    }
    frame #1 {
      w406 = dbl[] [-1.0]
      w477 = 0
      w452 = 0 ("Zyklusnummer1")
      n140 = while {
        tunnel: w430 -> [w860]
        tunnel: w499 -> [w859]
        tunnel: w498 -> [w858]
        tunnel: w497 -> [w857]
        shift-right: [w856] -> _
        shift-left: errorcluster {"status"=FALSE, "code"=0, "source"=""} ("error out") -> [w855]
        stop <- w861 stop-if-true
        n141 = call "AIsFIFORT-01-17.vi"("FPGA VI Reference In"=w860, "P2"=w859, "P1"=w858, "P0"=w857, "error in"=w855) -> ("error out"=w856:errorcluster)
        "AIsFIFOread" <- w856
        n142 = global read "gvbooleschRT.vi" "global stop RT"() -> (w861:bool)
      }
      n143 = Add Array Elements(numeric array=w426) -> (sum=w425:i32)
      n144 = Array Size(array=w434) -> (size(s)=w455:i32)
      n145 = Unbundle(w451) -> ("created path"=w450:path, "created path"=w448:path, "created path"=w447:path, "Dateiname Housekeeping"=w449:string, "DateinameECD1"=w446:string, "DateinameECD2"=w445:string, "tdms0"=w444:refnum<k34>, "tdms1"=w443:refnum<k34>, "tdms0"=w442:refnum<k34>, "tdms1"=w441:refnum<k34>, "tdms0"=w440:refnum<k34>, "tdms1"=w439:refnum<k34>)
      n146 = flat-sequence {
        frame #0 {
          n147 = control-ref of="graph"() -> (w504:refnum<vi>)
          n148 = control-ref of="manual control"() -> (w508:refnum<vi>)
          n149 = control-ref of="Licor-output"() -> (w507:refnum<vi>)
          n150 = control-ref of="Licor-parameter out"() -> (w506:refnum<vi>)
          n151 = call "licore (main).vi"(5:"Licor-parameter"=w506, "manual control"=w508, "raw data"=w507, 10:"Licor-parameter"="Licor-parameter out", "graph"=w504) -> ()  [unwired: 7 in]
        }
      }
      n152 = while {
        stop <- w1251 stop-if-true
        w1245 = 10.0
        n153 = call "Warten2"("Count(mSec)"=u32 1000) -> ()  [unwired: 1 out]
        n154 = global read "gvbooleschRT.vi" "global stop RT"() -> (w1251:bool)
        n155 = global read "GVTrapsMachs.vi" "Traps/Machs"() -> (w1241:dbl[])
        n156 = global read "GVAIs.vi" "AIs"() -> (w1242:dbl[])
        n157 = for {
          N: 9 -> [_]
          shift-right: [w1254] -> w1248
          shift-left: w1242 -> [w1255]
          shift-right: [w1252] -> w1246
          shift-left: w1241 -> [w1253]
          n158 = flat-sequence {
            tunnel: w1255 -> [w1262]
            tunnel: [w1261] -> w1254
            tunnel: w1253 -> [w1260]
            tunnel: [w1259] -> w1252
            frame #0 {
              n159 = call "Warten28"("Count(mSec)"=u32 100) -> ()  [unwired: 1 out]
            }
            frame #1 {
              n160 = global read "GVAIs.vi" "AIs"() -> (w1258:dbl[])
              n161 = Add(x=w1262, y=w1258) -> (x+y=w1261:dbl[])
              n162 = global read "GVTrapsMachs.vi" "Traps/Machs"() -> (w1257:dbl[])
              n163 = Add(x=w1257, y=w1260) -> (x+y=w1259:dbl[])
            }
          }
        }
        n164 = Divide(x=w1248, y=w1245) -> (x/y=w1247:dbl[])
        n165 = Divide(x=w1246, y=w1245) -> (x/y=w1244:dbl[])
        n166 = Build Array (concatenate)(w1247, w1244) -> (w1243:dbl[])
        n167 = global write "GVHK1Hz.vi" "Mod1Mod2Mod3/AITrapsMachs1Hz"(w1243) -> ()
      }
      n168 = while {
        shift-right: ["Methode"] -> _
        shift-left: w503 -> [w1265]
        stop <- w1267 stop-if-true
        n169 = call "Bis zum nächsten Vielfachen warten7"("Count(mSec)"=u32 1000) -> ()  [unwired: 1 out]
        n170 = Not Equal?(x=w1265, y="Methode") -> (x != y?=w1263:bool)
        n171 = global write "GVMethodenwechsel.vi" "Methodenwechsel?"(w1263) -> ()
        n172 = global read "gvbooleschRT.vi" "global stop RT"() -> (w1267:bool)
      }
      n173 = Index Array(array=w427, index #1=0 ("Index"), index #2=1 ("Index"), index #3=2 ("Index"), index #4=3 ("Index")) -> (element #1=w466:i32, element #2=w465:i32, element #3=w468:i32, element #4=w467:i32)
      n174 = while {
        tunnel: w430 -> [w862]
        tunnel: w405 -> [w867]
        tunnel: w404 -> [w866]
        tunnel: w403 -> [w865]
        shift-right: [w864] -> _
        shift-left: errorcluster {"status"=FALSE, "code"=0, "source"=""} ("error out") -> [w863]
        stop <- w869 stop-if-true
        n175 = call "TrapsMachMitteln-01-17.vi"("FPGA VI Reference In"=w862, "Traps/MachKoeff2"=w867, "Traps/MachKoeff1"=w866, "Traps/MachKoeff0"=w865, "error in"=w863) -> ("error out"=w864:errorcluster)
        "MWTrapsMachs" <- w864
        n176 = global read "gvbooleschRT.vi" "global stop RT"() -> (w869:bool)
        n177 = call "Bis zum nächsten Vielfachen warten16"("Count(mSec)"=u32 100) -> ()  [unwired: 1 out]
      }
      n178 = call <vilib>:"Space Constant.vi"() -> ("String"=w412:string)
      n179 = case shown="True" TRUE ("ECDSpeichern") {
        frame False {
        }
        frame True {
          w795 = dbl[] []
          n180 = global read "GVaktuelleTDMS.vi" "aktuelleTDMS-DateiECD1"() -> (w796:refnum<k34>)
          n181 = while {
            shift-right: [w808] -> _
            shift-left: w795 -> [w812]
            shift-right: [w801] -> _
            shift-left: w795 -> [w805]
            shift-right: [w807] -> _
            shift-left: w796 -> [w810]
            tunnel: w795 -> [w804]
            shift-right: [w798] -> _
            shift-left: errorcluster {"status"=FALSE, "code"=0, "source"=""} ("error IO") -> [w797]
            stop <- w817 stop-if-true
            n182 = global read "GVaktuelleTDMS.vi" "aktuelleTDMS-DateiECD1"() -> (w807:refnum<k34>)
            n183 = global read "GVaktuelleTDMS.vi" "aktuelleTDMS-DateiECD2"() -> (w815:refnum<k34>)
            n184 = call "Bis zum nächsten Vielfachen warten3"("Count(mSec)"=u32 500) -> ()  [unwired: 1 out]
            n185 = global read "GVECDs.vi" "ECD1MW"() -> (w811:dbl[])
            n186 = global read "GVECDs.vi" "ECD2MW"() -> (w802:dbl[])
            n187 = Equal?(x=w810, y=w807) -> (x = y?=w803:bool)
            n188 = Build Array (concatenate)(w812, w811) -> (w809:dbl[])
            n189 = Build Array (concatenate)(w805, w802) -> (w806:dbl[])
            n190 = TDMS Write(0:w807, 7:"ECD1", 9:w811, 11:w797) -> (15:w800:errorcluster)  [unwired: 2 in, 3 out]
            n191 = TDMS Write(0:w815, 7:"ECD2", 9:w802, 11:w797) -> (15:w799:errorcluster)  [unwired: 2 in, 3 out]
            n192 = Select(t=w806, s=w803, f=w804) -> (s? t:f=w801:dbl[])
            n193 = Select(t=w809, s=w803, f=w804) -> (s? t:f=w808:dbl[])
            n194 = Merge Errors(w800, w799) -> (w798:errorcluster)
            "TDMSwriteECD" <- w798
            n195 = global write "GVChroms.vi" "ECD2Chrom"(w801) -> ()
            n196 = global write "GVChroms.vi" "ECD1Chrom"(w808) -> ()
            n197 = global read "gvbooleschRT.vi" "global stop RT"() -> (w817:bool)
          }
        }
      }
      n198 = while {
        shift-right: [w511] -> _
        shift-left: w406 -> [w513]
        shift-right: [w510] -> _
        shift-left: w406 -> [w512]
        stop <- w515 stop-if-true
        n199 = call "Bis zum nächsten Vielfachen warten"("Count(mSec)"=u32 100) -> ()  [unwired: 1 out]
        n200 = case shown="True" "An/Aus" {
          tunnel: w513 -> [w517 w533]
          tunnel: w512 -> [w516 w532]
          tunnel: [w517 w526] -> w511
          tunnel: [w516 w525] -> w510
          frame False {
          }
          frame True {
            w529 = dbl[] [] ("t")
            n201 = global read "GVMWHorst.vi" "MWHorst"() -> (w522:dbl[])
            n202 = global read "GVTrapsMachs.vi" "Traps/Machs"() -> (w523:dbl[])
            n203 = Build Array (concatenate)(w523, w522) -> (w521:dbl[])
            n204 = Index Array(array=w521, index="dargestellte Größe 3") -> (element=w534:dbl)
            n205 = Build Array (concatenate)(w533, w534) -> (w527:dbl[])
            n206 = Select(t=w529, s="TafelWischen!", f=w527) -> (s? t:f=w526:dbl[])
            n207 = global read "GVZeitenZyklen.vi" "Big Ben, Methodenzeit, Zykluszeit0, Zykluszeit1, Zykluszeit2A, Zykluszeit2B"() -> (w520:dbl[])
            n208 = Index Array(array=w520, index=1 ("Index")) -> (element=w518:dbl)
            n209 = Build Array (concatenate)(w532, w518) -> (w528:dbl[])
            n210 = Select(t=w529, s="TafelWischen!", f=w528) -> (s? t:f=w525:dbl[])
            n211 = Bundle(w528, w527) -> (→"schnelleAnzeige":cluster{dbl[], dbl[]})  [unwired: 1 in]
          }
        }
        n212 = global read "gvbooleschRT.vi" "global stop RT"() -> (w515:bool)
      }
      n213 = case shown="True" TRUE ("HKSpeichern") {
        tunnel: w501 -> [_ w848]
        frame False {
        }
        frame True {
          n214 = while {
            tunnel: w848 -> [w852]
            shift-right: [w850] -> _
            shift-left: errorcluster {"status"=FALSE, "code"=0, "source"=""} ("error out") -> [w849]
            stop <- w854 stop-if-true
            n215 = local read "Methode"() -> (w851:i32)
            n216 = call "Bis zum nächsten Vielfachen warten2"("Count(mSec)"=u32 1000) -> ()  [unwired: 1 out]
            n217 = call "HKinTDMS-01-16.vi"("Methode"=w851, "error in (no error)"=w849, "Kanäle"=w852) -> ("error out"=w850:errorcluster)
            "TDMSwriteHK" <- w850
            n218 = global read "gvbooleschRT.vi" "global stop RT"() -> (w854:bool)
          }
        }
      }
      n219 = for {
        N: 1 -> [_]
        tunnel: w430 -> [w870]
        tunnel: [w870] -> w457
        n220 = call "Warten8"("Count(mSec)"=u32 100) -> ()  [unwired: 1 out]
      }
      n221 = global read "GVVentilposition.vi" "Ventilposition"() -> (w436:i32)
      n222 = Build Array(w412) -> (w411:string[])
      n223 = Initialize Array(-1 ("Element"), 4 ("Dimension")) -> (w428:i32[])
      n224 = case shown="True" TRUE {
        tunnel: w452 -> [_ w827]
        tunnel: w450 -> [_ w826]
        tunnel: w449 -> [_ w825]
        tunnel: w444 -> [_ w824]
        tunnel: w443 -> [_ w823]
        frame False {
        }
        frame True {
          w818 = errorcluster {"status"=FALSE, "code"=0, "source"=""} ("error out TDMSopen")
          n225 = while {
            shift-right: [w832] -> w822
            shift-left: w824 -> [w834]
            shift-right: [w843] -> w821
            shift-left: w823 -> [w836]
            shift-right: [w838] -> _
            shift-left: w827 -> [w844]
            tunnel: w825 -> [w840]
            tunnel: w826 -> [w841]
            shift-right: [w831] -> w820
            shift-left: w818 -> [w829]
            shift-right: [w830] -> w819
            shift-left: w818 -> [w828]
            stop <- w846 stop-if-true
            n226 = global read "GVZeitenZyklen.vi" "ZyklusNummernGesamt"() -> (w833:i32[])
            n227 = call "Bis zum nächsten Vielfachen warten5"("Count(mSec)"=u32 500) -> ()  [unwired: 1 out]
            n228 = Index Array(array=w833, index=1 ("Index")) -> (element=w838:i32)
            n229 = Greater?(x=w838, y=w844) -> (0:w837:bool)
            n230 = Select(t=w836, s=w837, f=w834) -> (s? t:f=w835:refnum<k34>)
            n231 = local read "Methode"() -> (w842:i32)
            n232 = global write "GVaktuelleTDMS.vi" "aktuelleTDMS-DateiHK"(w835) -> ()
            n233 = call "AktuelleTDMS.vi"("AktuelleTDMS"=w834, "error in TDMSopen"=w829, "Dateiordner"=w841, "NächsteTDMS"=w836, "NeuerZyklus?"=w837, "Methodennummer"=w842, "Zyklnumges"=w838, "error in TDMSclose"=w828, "Dateiname"=w840) -> ("AktuelleTDMS"=w832:refnum<k34>, "error out TDMSopen"=w831:errorcluster, "error out TDMSclose"=w830:errorcluster, "NächsteTDMS"=w843:refnum<k34>)  [unwired: 3 in]
            "TDMSopenHK" <- w831
            "TDMScloseHK" <- w830
            n234 = global read "gvbooleschRT.vi" "global stop RT"() -> (w846:bool)
          }
          n235 = TDMS Close(8:w820, 11:w822) -> ()  [unwired: 2 out]
          n236 = TDMS Close(8:w819, 11:w821) -> ()  [unwired: 2 out]
        }
      }
      n237 = case shown="True" TRUE {
        tunnel: w452 -> [_ w755]
        tunnel: w448 -> [_ w754]
        tunnel: w447 -> [_ w753]
        tunnel: w446 -> [_ w752]
        tunnel: w445 -> [_ w751]
        tunnel: w442 -> [_ w750]
        tunnel: w441 -> [_ w749]
        tunnel: w440 -> [_ w748]
        tunnel: w439 -> [_ w747]
        frame False {
        }
        frame True {
          w740 = errorcluster {"status"=FALSE, "code"=0, "source"=""} ("error out TDMSopen")
          n238 = while {
            shift-right: [w779] -> w746
            shift-left: w750 -> [w781]
            shift-right: [w789] -> w745
            shift-left: w749 -> [w783]
            shift-right: [w787] -> _
            shift-left: w755 -> [w790]
            tunnel: w754 -> [w786]
            tunnel: w752 -> [w785]
            shift-right: [w778] -> w741
            shift-left: w740 -> [w776]
            shift-right: [w777] -> w742
            shift-left: w740 -> [w775]
            stop <- w792 stop-if-true
            n239 = global read "GVZeitenZyklen.vi" "ZyklusNummernGesamt"() -> (w780:i32[])
            n240 = call "Bis zum nächsten Vielfachen warten4"("Count(mSec)"=u32 500) -> ()  [unwired: 1 out]
            n241 = Index Array(array=w780, index=2 ("Index")) -> (element=w787:i32)
            n242 = Greater?(x=w787, y=w790) -> (0:w784:bool)
            n243 = Select(t=w783, s=w784, f=w781) -> (s? t:f=w782:refnum<k34>)
            n244 = local read "Methode"() -> (w788:i32)
            n245 = global write "GVaktuelleTDMS.vi" "aktuelleTDMS-DateiECD1"(w782) -> ()
            n246 = call "AktuelleTDMS.vi"("AktuelleTDMS"=w781, "error in TDMSopen"=w776, "Dateiordner"=w786, "NächsteTDMS"=w783, "NeuerZyklus?"=w784, "Methodennummer"=w788, "Zyklnumges"=w787, "error in TDMSclose"=w775, "Dateiname"=w785) -> ("AktuelleTDMS"=w779:refnum<k34>, "error out TDMSopen"=w778:errorcluster, "error out TDMSclose"=w777:errorcluster, "NächsteTDMS"=w789:refnum<k34>)  [unwired: 3 in]
            "TDMSopenECD1" <- w778
            "TDMScloseECD1" <- w777
            n247 = global read "gvbooleschRT.vi" "global stop RT"() -> (w792:bool)
          }
          n248 = while {
            shift-right: [w769] -> w744
            shift-left: w748 -> [w761]
            shift-right: [w770] -> w743
            shift-left: w747 -> [w763]
            shift-right: [w767] -> _
            shift-left: w755 -> [w771]
            tunnel: w753 -> [w766]
            tunnel: w751 -> [w765]
            shift-right: [w759] -> _
            shift-left: w740 -> [w757]
            shift-right: [w758] -> _
            shift-left: w740 -> [w756]
            stop <- w773 stop-if-true
            n249 = global read "GVZeitenZyklen.vi" "ZyklusNummernGesamt"() -> (w760:i32[])
            n250 = call "Bis zum nächsten Vielfachen warten6"("Count(mSec)"=u32 500) -> ()  [unwired: 1 out]
            n251 = Index Array(array=w760, index=3 ("Index")) -> (element=w767:i32)
            n252 = Greater?(x=w767, y=w771) -> (0:w764:bool)
            n253 = Select(t=w763, s=w764, f=w761) -> (s? t:f=w762:refnum<k34>)
            n254 = local read "Methode"() -> (w768:i32)
            n255 = global write "GVaktuelleTDMS.vi" "aktuelleTDMS-DateiECD2"(w762) -> ()
            n256 = call "AktuelleTDMS.vi"("AktuelleTDMS"=w761, "error in TDMSopen"=w757, "Dateiordner"=w766, "NächsteTDMS"=w763, "NeuerZyklus?"=w764, "Methodennummer"=w768, "Zyklnumges"=w767, "error in TDMSclose"=w756, "Dateiname"=w765) -> ("AktuelleTDMS"=w769:refnum<k34>, "error out TDMSopen"=w759:errorcluster, "error out TDMSclose"=w758:errorcluster, "NächsteTDMS"=w770:refnum<k34>)  [unwired: 3 in]
            "TDMSopenECD2" <- w759
            "TDMScloseECD2" <- w758
            n257 = global read "gvbooleschRT.vi" "global stop RT"() -> (w773:bool)
          }
          n258 = TDMS Close(8:w741, 11:w746) -> ()  [unwired: 2 out]
          n259 = TDMS Close(8:w742, 11:w745) -> ()  [unwired: 2 out]
          n260 = TDMS Close(11:w744) -> ()  [unwired: 1 in, 2 out]
          n261 = TDMS Close(11:w743) -> ()  [unwired: 1 in, 2 out]
        }
      }
      n262 = Add(x=w468, y=w467) -> (x+y=w464:i32)
      n263 = Bundle(w411, w411, w411) -> (w475:cluster{string[], string[], string[]})  [unwired: 1 in]
      n264 = Index Array(array=w421, index=w419) -> (element=w420:T15)
      n265 = Initialize Array(cluster{"output high":dbl, "output low":dbl} {"output high"=99999.0, "output low"=0.0} ("output range"), w455) -> (w435:cluster{"output high":dbl, "output low":dbl}[])
      n266 = Concatenate Strings("?SE0,GDATA" ("Schreibpuffer"), "\r") -> (w407:string)
      n267 = Build Array(w466, w465, w464) -> (w463:i32[])
      n268 = while {
        tunnel: w502 -> [w996]
        shift-right: [w995] -> _
        shift-left: w421 -> [w977]
        tunnel: w435 -> [w994]
        tunnel: w434 -> [w993]
        tunnel: w430 -> [w992]
        tunnel: w433 -> [w991]
        tunnel: w432 -> [w990]
        shift-right: [w984] -> _
        shift-left: 0 -> [w989]
        tunnel: w430 -> [w988]
        tunnel: w429 -> [w987]
        shift-right: [w983] -> _
        shift-left: w428 -> [w986]
        tunnel: w427 -> [w978]
        tunnel: w426 -> [w979]
        tunnel: w425 -> [w980]
        tunnel: w424 -> [w981]
        tunnel: w423 -> [w982]
        tunnel: w422 -> [w985]
        shift-right: [w900] -> _
        shift-left: w420 -> [w899]
        tunnel: w405 -> [w878]
        tunnel: w404 -> [w882]
        tunnel: w403 -> [w888]
        i -> [w903]
        stop <- w997 stop-if-true
        w889 = 0  # ZeileMainMach2
        w890 = 0  # ZeileMainMach1
        w945 = FALSE
        w944 = 0.0
        w946 = 0  # ZeilennummerMPV
        w950 = cluster{dbl[], dbl[]} {[], []}
        w959 = dbl[] []
        w963 = 0  # ZeilePreMach2
        w964 = 0  # ZeilePreMach1
        w965 = 0  # ZeileFPGAFixp
        w966 = 0  # ZeileFPGAPID
        w967 = 0  # ZeileFPGABoolesch
        w968 = i32[] [0, 0, 0, 0]  # ZeilennummernHorst
        w969 = i32[] [0, 0, 0, 0]  # ZeilennummernDIOs
        n269 = Unbundle(w899) -> ("Zykluslängen [s]"=w943:dbl[], "ZeitpktDIOsMod0"=w942:dbl[], "ZeitpktDIOsMod1"=w941:dbl[], "ZeitpktDIOsMod2A"=w940:dbl[], "ZeitpktDIOsMod2B"=w939:dbl[], "DIOsSPMod0"=w938:bool[][], "DIOsSPMod1"=w937:bool[][], "DIOsSPMod2A"=w936:bool[][], "DIOsSPMod2B"=w935:bool[][], "Mod0HorstZeitpkt"=w934:dbl[], "Mod1HorstZeitpkt"=w933:dbl[], "Mod2AHorstZeitpkt"=w932:dbl[], "Mod2BHorstZeitpkt"=w931:dbl[], "HorstSPMod0"=w930:dbl[][], "HorstSPMod1"=w929:dbl[][], "HorstSPMod2A"=w928:dbl[][], "HorstSPMod2B"=w927:dbl[][], "LHSetpoints"=w926:dbl[], "LHHeizen?"=w925:bool[], "ZPktFPGABoolesch"=w924:dbl[], "FPGABoolesch"=w923:bool[][], "ZeitpktFPGAPID"=w922:dbl[], "FPGAPID"=w921:T17, "ZeitpktFPGAFixp"=w920:dbl[], "SHSetpoints"=w919:dbl[][], "t_PreMach1"=w918:dbl[], "T_PreMach1"=w917:dbl[], "t_PreMach2"=w916:dbl[], "T_PreMach2"=w915:dbl[], "PIDs für \"träge\" Heizungen"=w914:T18, "Zwangsbedingungen"=w913:dbl[][], "Dateien fürs MS schicken?"=w912:bool, "ZeitpunkteMPV"=w911:dbl[], "SPMPV"=w910:i32[], "ZeitpktMS-1"=w909:dbl, "ZeitpktMS-2"=w908:dbl, "Int.Start1"=w907:dbl, "Int.Stop1"=w906:dbl, "Int.Start2"=w905:dbl, "Int.Stop2"=w904:dbl, "t_MainMach1"=w898:dbl[], "T_MainMach1"=w897:dbl[], "t_MainMach2"=w896:dbl[], "T_MainMach2"=w895:dbl[])  [unwired: 1 out]
        n270 = Add(x=w986, y=1) -> (x+y=w954:i32[])
        n271 = Array Subset(array=w888, index=2 ("Index"), length=4 ("Länge")) -> (w885:dbl[])
        n272 = Array Subset(array=w882, index=2 ("Index"), length=4 ("Länge")) -> (w881:dbl[])
        n273 = Array Subset(array=w878, index=2 ("Index"), length=4 ("Länge")) -> (w877:dbl[])
        n274 = local read "Methode"() -> (w902:i32)
        n275 = while {
          tunnel: w979 -> [w1070]
          tunnel: w982 -> [w1068]
          tunnel: w981 -> [w1067]
          tunnel: w978 -> [w1069]
          tunnel: w980 -> [w1066]
          tunnel: w913 -> [w1058]
          stop <- w1060 stop-if-true
          n276 = call "Bis zum nächsten Vielfachen warten10"("Count(mSec)"=u32 1000) -> ()  [unwired: 1 out]
          n277 = local read "Methode"() -> (w1065:i32)
          n278 = global read "GVMethodenwechsel.vi" "Methodenwechsel?"() -> (w1062:bool)
          n279 = global read "gvbooleschRT.vi" "global stop RT"() -> (w1063:bool)
          n280 = case shown="True" "global stop RT" {
            frame False {
            }
            frame True {
              n281 = global write "gvbooleschRT.vi" "global stop RT"(TRUE ("global stop RT")) -> ()
            }
          }
          n282 = call "ZwangsbedingungenGV.vi"("AnzahlHorst"=w1068, "AnzahlHorst/Modul"=w1069, "AnzahlLH"=w1067, "AnzahlDIOs/Modul"=w1070, "AnzahlDIOs"=w1066, "Zwangsbedingungen"=w1058, "Methodennummer"=w1065) -> ("Methodennummer"=w1064:i32)  [unwired: 4 in]
          n283 = local write "Methode"(w1064) -> ()
          n284 = local read "veränderte Methode benutzen"() -> (w1061:bool)
          n285 = Compound Arithmetic op=OR(w1063, w1062, w1061) -> (w1060:bool)
        }
        n286 = while {
          tunnel: w993 -> [w1049]
          tunnel: w994 -> [w1051]
          tunnel: w992 -> [w1046]
          tunnel: w926 -> [w1050]
          tunnel: w914 -> [w1052]
          shift-right: [w1048] -> _
          shift-left: errorcluster {"status"=FALSE, "code"=0, "source"=""} ("error out") -> [w1047]
          stop <- w1053 stop-if-true
          n287 = call "LH-01-17.vi"("FPGA VI Reference In"=w1046, "OutputRange"=w1051, "LHSetpoints"=w1050, "AIsLH"=w1049, "error in"=w1047, "PIDs für \"träge\" Heizungen"=w1052) -> ("error out"=w1048:errorcluster)  [unwired: 1 in]
          "LH" <- w1048
          n288 = call "Bis zum nächsten Vielfachen warten12"("Count(mSec)"=u32 100) -> ()  [unwired: 1 out]
          n289 = local read "veränderte Methode benutzen"() -> (w1054:bool)
          n290 = global read "GVMethodenwechsel.vi" "Methodenwechsel?"() -> (w1055:bool)
          n291 = global read "gvbooleschRT.vi" "global stop RT"() -> (w1056:bool)
          n292 = Compound Arithmetic op=OR(w1056, w1055, w1054) -> (w1053:bool)
        }
        n293 = Build Cluster Array(w938, w937, w936, w935) -> (w973:cluster{"DIOsSPMod2B":bool[][]}[])
        n294 = Build Cluster Array(w930, w929, w928, w927) -> (w971:cluster{"HorstSPMod2B":dbl[][]}[])
        n295 = Build Cluster Array(w942, w941, w940, w939) -> (w974:cluster{"ZeitpktDIOsMod2B":dbl[]}[])
        n296 = Build Cluster Array(w934, w933, w932, w931) -> (w972:cluster{"Mod2BHorstZeitpkt":dbl[]}[])
        n297 = Bundle(w885, w881, w877) -> (w876:cluster{dbl[], dbl[], dbl[]})  [unwired: 1 in]
        n298 = Equal?(x=w903, y=0) -> (x = y?=w975:bool)
        n299 = global read "GVZeitenZyklen.vi" "ZyklusNummern"() -> (w953:i32[])
        n300 = global read "GVZwangs.vi" "ZwangsHorst?"() -> (w958:cluster{bool[]}[])
        n301 = global read "gvbooleschRT.vi" "global stop RT"() -> (w997:bool)
        n302 = global read "GVZwangsMPV.vi" "ZwangsMPV?"() -> (w874:bool)
        n303 = global read "GVZwangs.vi" "ZwangsDIO?"() -> (w957:cluster{bool[]}[])
        n304 = global read "GVaktuelleTDMS.vi" "aktuelleTDMS-DateiECD1"() -> (w952:refnum<k34>)
        n305 = global read "GVZwangs.vi" "ZwangsFPGABoolesch?"() -> (w956:bool[])
        n306 = while {
          shift-right: [w1010] -> _
          shift-left: w945 -> [w1014]
          shift-right: [w1009] -> _
          shift-left: w944 -> [w1013]
          shift-right: [w1008] -> _
          shift-left: w945 -> [w1012]
          shift-right: [w1007] -> _
          shift-left: w944 -> [w1011]
          tunnel: w985 -> [w1006]
          tunnel: w907 -> [w1001]
          tunnel: w906 -> [w1000]
          tunnel: w905 -> [w999]
          tunnel: w904 -> [w998]
          stop <- w1003 stop-if-true
          n307 = call "Integrieren.vi"("Integrieren1"=w1014, "Integral1"=w1013, "Integrieren2"=w1012, "Integral2"=w1011, "Int.Start1"=w1001, "Int.Stop1"=w1000, "Int.Start2"=w999, "HorstProbenflußNr."=w1006, "Int.Stop2"=w998) -> ("Integrieren1"=w1010:bool, "Integral1"=w1009:dbl, "Integrieren2"=w1008:bool, "Integral2"=w1007:dbl)  [unwired: 7 in]
          n308 = call "Bis zum nächsten Vielfachen warten9"("Count(mSec)"=u32 100) -> ()  [unwired: 1 out]
          n309 = global read "GVMethodenwechsel.vi" "Methodenwechsel?"() -> (w1004:bool)
          n310 = global read "gvbooleschRT.vi" "global stop RT"() -> (w1005:bool)
          n311 = local read "veränderte Methode benutzen"() -> (w1002:bool)
          n312 = Compound Arithmetic op=OR(w1005, w1004, w1002) -> (w1003:bool)
        }
        n313 = while "Zeit" {
          tunnel: w975 -> [w1202]
          tunnel: w943 -> [w1200]
          tunnel: w954 -> [w1195]
          tunnel: [w1194] -> w983
          shift-right: [w1191] -> _
          shift-left: 0.0 -> [w1192]
          i -> [w1204]
          stop <- w1197 stop-if-true
          n314 = Equal?(x=w1204, y=0) -> (x = y?=w1193:bool)
          n315 = call "Bis zum nächsten Vielfachen warten15"("Count(mSec)"=u32 50) -> ()  [unwired: 1 out]
          n316 = call "BigBen-01-16.vi"("MethodenStartzeit"=w1192, "Methodenstart?"=w1193, "Programmstart?"=w1202, "Zykluslängen [s]"=w1200, "MethodenStartZyklusNummern"=w1195) -> ("MethodenStartzeit"=w1191:dbl, "ZyklusNummernGesamt"=w1194:i32[])  [unwired: 2 in]
          n317 = global read "GVMethodenwechsel.vi" "Methodenwechsel?"() -> (w1196:bool)
          n318 = global read "gvbooleschRT.vi" "global stop RT"() -> (w1201:bool)
          n319 = local read "veränderte Methode benutzen"() -> (w1199:bool)
          n320 = Or(x=w1196, y=w1201) -> (x .or. y?=w1198:bool)
          n321 = Or(x=w1199, y=w1198) -> (x .or. y?=w1197:bool)
        }
        n322 = Bundle(w974, w973, w972, w971, "LHHeizen?"=w925, "ZPktFPGABoolesch"=w924, "FPGABoolesch"=w923, "ZeitpktFPGAPID"=w922, "FPGAPID"=w921, "ZeitpktFPGAFixp"=w920, "SHSetpoints"=w919, "t_PreMach1"=w918, "T_PreMach1"=w917, "t_PreMach2"=w916, "T_PreMach2"=w915, "ZeitpunkteMPV"=w911, "SPMPV"=w910, "t_MainMach1"=w898, "T_MainMach1"=w897, "t_MainMach2"=w896, "T_MainMach2"=w895) -> (w970:T19)  [unwired: 1 in]
        n323 = Index Array(array=w977, index=w902) -> (element=w901:T15)
        n324 = while {
          tunnel: w996 -> [w1217]
          shift-right: [w1208] -> _
          shift-left: w901 -> [w1216]
          tunnel: w902 -> [w1214]
          shift-right: [w1206] -> w995
          shift-left: w977 -> [w1215]
          tunnel: [w1207] -> w900
          stop <- w1210 stop-if-true
          n325 = call "Bis zum nächsten Vielfachen warten8"("Count(mSec)"=u32 500) -> ()  [unwired: 1 out]
          n326 = global read "GVMethodenwechsel.vi" "Methodenwechsel?"() -> (w1212:bool)
          n327 = global read "gvbooleschRT.vi" "global stop RT"() -> (w1211:bool)
          n328 = case shown="True" "Methode verändern" {
            tunnel: w1217 -> [_ w1239]
            tunnel: w1216 -> [w1236 w1238]
            tunnel: [w1236 w1237] -> w1208
            frame False {
            }
            frame True {
              n329 = call "methodeändern-11-15.vi"("Methode"=w1238, "Namen"=w1239) -> ("Methode"=w1237:T20)  [unwired: 1 in]
              n330 = property on="Methode verändern" class="Bool (strict)"("Value"=FALSE ("Methode verändern")) -> ()  [unwired: 2 in, 2 out]
            }
          }
          n331 = Compound Arithmetic op=OR(w1212, w1211, "veränderte Methode benutzen") -> (w1210:bool)
          n332 = case shown="True" "Methode speichern" {
            tunnel: w1208 -> [_ w1233]
            tunnel: w1215 -> [w1226 w1235]
            tunnel: w1214 -> [_ w1234]
            tunnel: [w1226 w1228] -> w1206
            frame False {
            }
            frame True {
              n333 = Replace Array Subset(array=w1235, new element=w1233, index=w1234) -> (w1228:T9)
              n334 = property on="Methode speichern" class="Bool (strict)"("Value"=FALSE ("Methode speichern")) -> ()  [unwired: 2 in, 2 out]
              n335 = Open/Create/Replace File(file path (use dialog)=path "c:/methoden.per" ("Dateipfad (Dialog verwenden)"), operation (0:open)=T10."replace" ("Operation (0:Öffnen)")) -> (refnum out=w1230:refnum<file>)  [unwired: 4 in, 2 out]
              n336 = Write to Binary File(file (use dialog)=w1230, data=w1228) -> (refnum out=w1227:refnum<file>)  [unwired: 4 in, 2 out]
              n337 = Close File(refnum=w1227) -> ()  [unwired: 1 in, 2 out]
            }
          }
          n338 = case shown="False" "veränderte Methode benutzen" {
            tunnel: w1208 -> [_ w1223]
            tunnel: [w1220 w1223] -> w1207
            tunnel: w1206 -> [w1222 _]
            frame False {
              n339 = local read "Methode"() -> (w1221:i32)
              n340 = Index Array(array=w1222, index=w1221) -> (element=w1220:T15)
            }
            frame True {
              n341 = flat-sequence {
                frame #0 {
                  n342 = call "Warten"("Count(mSec)"=u32 1100) -> ()  [unwired: 1 out]
                }
                frame #1 {
                  n343 = property on="veränderte Methode benutzen" class="Bool (strict)"("Value"=FALSE ("Methode verändern")) -> ()  [unwired: 2 in, 2 out]
                }
              }
            }
          }
        }
        n344 = Bundle(w959, w959, w959, w959) -> (w960:cluster{dbl[], dbl[], dbl[], dbl[]})  [unwired: 1 in]
        n345 = Bundle("ZyklusNummern"=w953, "ZeilennummernDIOs"=w969, "ZwangsDIO?"=w957, "ZeilennummernHorst"=w968, "ZwangsHorst?"=w958, "ZeileFPGABoolesch"=w967, "ZwangsFPGABoolesch?"=w956, "ZeileFPGAPID"=w966, "ZeileFPGAFixp"=w965, "ZeilePreMach1"=w964, "ZeilePreMach2"=w963, "ZeilennummerMPV"=w946, "ZeileMainMach1"=w890, "ZeileMainMach2"=w889, "ZwangsMPV?"=w874) -> (w962:T21)  [unwired: 1 in]
        n346 = call "arrayDoppelMoppel-11-15.vi"("verdoppeln"=i32[] [0, 1], "Traps/MachsKoeff2"=w878, "Traps/MachsKoeff1"=w882, "Traps/MachsKoeff0"=w888) -> ("Traps/MachsKoeff2"=w891:dbl[], "Traps/MachsKoeff1"=w892:dbl[], "Traps/MachsKoeff0"=w893:dbl[])  [unwired: 5 in]
        n347 = while "ZyklusSteuerung" {
          tunnel: w987 -> [w1184]
          tunnel: w988 -> [w1174]
          shift-right: [w1183] -> _
          shift-left: w962 -> [w1177]
          tunnel: w970 -> [w1181]
          tunnel: w893 -> [w1180]
          tunnel: w892 -> [w1179]
          tunnel: w891 -> [w1178]
          tunnel: w876 -> [w1182]
          shift-right: [w1176] -> _
          shift-left: errorcluster {"status"=FALSE, "code"=0, "source"=""} ("error out") -> [w1175]
          stop <- w1186 stop-if-true
          n348 = local read "veränderte Methode benutzen"() -> (w1187:bool)
          n349 = call "Bis zum nächsten Vielfachen warten11"("Count(mSec)"=u32 100) -> ()  [unwired: 1 out]
          n350 = global read "GVMethodenwechsel.vi" "Methodenwechsel?"() -> (w1189:bool)
          n351 = global read "gvbooleschRT.vi" "global stop RT"() -> (w1188:bool)
          n352 = call "ZyklussteuerungGV-01-17.vi"("Traps/MachKoeff0"=w1180, "DIOsNummern"=w1184, "error in"=w1175, "Traps/MachKoeff1"=w1179, "ServosWarmHigh (us)KaltHigh(us)"="ServosWarmHigh (us)KaltHigh(us)", "Traps/MachKoeff2"=w1178, "Schieberegister"=w1177, "Zeitpunkte/Setpoints"=w1181, "FPGA VI Reference In"=w1174, "MachKoeffs"=w1182) -> ("Schieberegister"=w1183:T22, "error out"=w1176:errorcluster)  [unwired: 4 in]
          "Zyklus" <- w1176
          n353 = Compound Arithmetic op=OR(w1189, w1188, w1187) -> (w1186:bool)
        }
        n354 = while {
          shift-right: [w1122] -> _
          shift-left: w960 -> [w1129]
          shift-right: [w1121] -> _
          shift-left: w960 -> [w1128]
          shift-right: [w1119] -> _
          shift-left: T13 {"Zyklus1"=0, "Zeitachse1"=0, "dargestellte Größe 1"=0, "Zyklus2"=0, "Zeitachse2"=0, "dargestellte Größe 2"=0} ("AnzeigeEinstellungen") -> [w1127]
          tunnel: w943 -> [w1097]
          shift-right: [w1093] -> _
          shift-left: w952 -> [w1092]
          shift-right: [w1088] -> _
          shift-left: w950 -> [w1090]
          shift-right: [w1077] -> _
          shift-left: w950 -> [w1089]
          shift-right: ["Detektor"] -> _
          shift-left: 0 ("Detektor") -> [w1086]
          stop <- w1133 stop-if-true
          w1098 = 0.0 ("X-Achse.Bereich:Minimum")
          n355 = call "Bis zum nächsten Vielfachen warten14"("Count(mSec)"=u32 1000) -> ()  [unwired: 1 out]
          n356 = global read "GVMWHorst.vi" "MWHorst"() -> (→"MWHorst":dbl[])
          n357 = case shown="True" TRUE ("Tabellarische Darstellung") {
            frame False {
            }
            frame True {
              n358 = global read "GVHK1Hz.vi" "Mod1Mod2Mod3/AITrapsMachs1Hz"() -> (w1139:dbl[])
              n359 = Array Subset(array=w1139, index=0 ("Index"), length=32 ("Länge")) -> (→"AIs1":dbl[])
              n360 = Array Subset(array=w1139, index=32 ("Index"), length=32 ("Länge")) -> (→"AIs2":dbl[])
              n361 = Array Subset(array=w1139, index=64 ("Index"), length=32 ("Länge")) -> (→"AIs3":dbl[])
            }
          }
          n362 = case shown="0, Default" "Detektor" {
            tunnel: [w1153 w1165] -> w1088
            tunnel: w1097 -> [w1152 w1167]
            tunnel: "Detektor" -> [w1147 w1161]
            tunnel: [w1151 w1166] -> w1095
            tunnel: [w1150 w1164] -> w1093
            frame 0, Default {
              n363 = Increment(x=w1147) -> (x+1=w1148:i32)
              n364 = Increment(x=w1148) -> (x+1=w1146:i32)
              n365 = global read "GVChroms.vi" "ECD1Chrom"() -> (w1149:dbl[])
              n366 = global read "GVaktuelleTDMS.vi" "aktuelleTDMS-DateiECD1"() -> (w1150:refnum<k34>)
              n367 = Index Array(array=w1152, index=w1146) -> (element=w1151:dbl)
              n368 = Array Size(array=w1149) -> (size(s)=w1155:i32)
              n369 = for {
                N: w1155 -> [_]
                tunnel: [w1156] -> w1154 mode=indexing
                i -> [w1159]
                n370 = To Double Precision Float(number=w1159) -> (double precision float=w1158:dbl)
                n371 = Divide(x=w1158, y=10.0) -> (x/y=w1156:dbl)
              }
              n372 = Bundle(w1154, "ECD1Chrom"=w1149) -> (w1153:cluster{dbl[], "ECD1Chrom":dbl[]})  [unwired: 1 in]
            }
            frame 1 {
              n373 = Increment(x=w1161) -> (x+1=w1162:i32)
              n374 = Increment(x=w1162) -> (x+1=w1160:i32)
              n375 = global read "GVChroms.vi" "ECD2Chrom"() -> (w1163:dbl[])
              n376 = global read "GVaktuelleTDMS.vi" "aktuelleTDMS-DateiECD2"() -> (w1164:refnum<k34>)
              n377 = Index Array(array=w1167, index=w1160) -> (element=w1166:dbl)
              n378 = Array Size(array=w1163) -> (size(s)=w1169:i32)
              n379 = for {
                N: w1169 -> [_]
                tunnel: [w1170] -> w1168 mode=indexing
                i -> [w1173]
                n380 = To Double Precision Float(number=w1173) -> (double precision float=w1172:dbl)
                n381 = Divide(x=w1172, y=10.0) -> (x/y=w1170:dbl)
              }
              n382 = Bundle(w1168, "ECD2Chrom"=w1163) -> (w1165:cluster{dbl[], "ECD2Chrom":dbl[]})  [unwired: 1 in]
            }
          }
          n383 = Equal?(x="Detektor", y=w1086) -> (x = y?=w1085:bool)
          n384 = Subtract(x="HK1YMax", y="HK1YMin") -> (x-y=w1113:dbl)
          n385 = Subtract(x="HK2YMax", y="HK2YMin") -> (x-y=w1108:dbl)
          n386 = Subtract(x="DetYMax", y="DetYMin") -> (x-y=w1103:dbl)
          n387 = global read "GVMethodenwechsel.vi" "Methodenwechsel?"() -> (w1131:bool)
          n388 = global read "GVZeitenZyklen.vi" "ZyklusNummern"() -> (w1100:i32[])
          "ZyklusNummern" <- w1100
          n389 = global read "GVMetavariablen.vi" "Metavariablen"() -> (→"Metavariablen":dbl[])
          n390 = global read "gvbooleschRT.vi" "global stop RT"() -> (w1132:bool)
          n391 = global read "GVVentilposition.vi" "Ventilposition"() -> (→"Ventilposition":i32)
          n392 = Divide(x=w1113, y=10.0) -> (x/y=w1111:dbl)
          n393 = Divide(x=w1108, y=10.0) -> (x/y=w1106:dbl)
          n394 = Divide(x=w1103, y=20.0) -> (x/y=w1101:dbl)
          n395 = global read "GVZeitenZyklen.vi" "ZyklusNummernGesamt"() -> (→"ZyklusNummernGesamt":i32[])
          n396 = local read "veränderte Methode benutzen"() -> (w1130:bool)
          n397 = Or(x=w1131, y=w1132) -> (x .or. y?=w1134:bool)
          n398 = global read "GVZeitenZyklen.vi" "Big Ben, Methodenzeit, Zykluszeit0, Zykluszeit1, Zykluszeit2A, Zykluszeit2B"() -> (w1080:dbl[])
          n399 = Or(x=w1134, y=w1130) -> (x .or. y?=w1133:bool)
          n400 = To Long Integer(number=w1080) -> (32bit integer=→"Big Ben, Methodenzeit, Zykluszeit0, Zykluszeit1, Zykluszeit2A, Zykluszeit2B":i32[])
          n401 = Equal?(x=w1093, y=w1092) -> (x = y?=w1091:bool)
          n402 = call "AnzeigeGV.vi"("veränderte Methode benutzen"=w1130, "Zykluslängen [s]"=w1097, "Cluster1"=w1129, "Big Ben, Methodenzeit, Zykluszeit0, Zykluszeit1, Zykluszeit2A, Zykluszeit2B"=w1080, "Zyklusnummern 0, 1, 2A, 2B"=w1100, "Cluster2"=w1128, "AnzeigeEinstellungen"=w1127, "dargestellte Größe 1"="dargestellte Größe 1", "Zeitachse1"="Zeitachse1", "dargestellte Größe 2"="dargestellte Größe 2", "Zeitachse2"="Zeitachse2") -> ("Anzeige2"=→"Housekeeping2":cluster{dbl[], dbl[]}, "Cluster1"=w1122:cluster{dbl[], dbl[], dbl[], dbl[]}, "x1Inkr"=w1117:dbl, "Cluster2"=w1121:cluster{dbl[], dbl[], dbl[], dbl[]}, "Anzeige1"=→"Housekeeping1":cluster{dbl[], dbl[]}, "AnzeigeEinstellungen"=w1119:T13, "x2Max"=w1081:dbl, "x2Inkr"=w1116:dbl, "x1Max"=w1082:dbl)  [unwired: 8 in]
          n403 = Divide(x=w1095, y=20.0) -> (x/y=w1096:dbl)
          n404 = Select(t=w1089, s=w1091, f=w1090) -> (s? t:f=w1084:cluster{dbl[], dbl[]})
          n405 = property on="Housekeeping1" class="XYGraph (strict)"("XScale.Minimum"=w1098, "XScale.Maximum"=w1082, "XScale.Increment"=w1117, "YScale.Minimum"="HK1YMin", "YScale.Maximum"="HK1YMax", "YScale.Increment"=w1111) -> ()  [unwired: 2 in, 2 out]
          n406 = property on="Housekeeping2" class="XYGraph (strict)"("XScale.Minimum"=w1098, "XScale.Maximum"=w1081, "XScale.Increment"=w1116, "YScale.Minimum"="HK2YMin", "YScale.Maximum"="HK2YMax", "YScale.Increment"=w1106) -> ()  [unwired: 2 in, 2 out]
          n407 = property on="Detektor 2" class="XYGraph (strict)"("XScale.Minimum"=w1098, "XScale.Maximum"=w1095, "XScale.Increment"=w1096, "YScale.Minimum"="DetYMin", "YScale.Maximum"="DetYMax", "YScale.Increment"=w1101) -> ()  [unwired: 2 in, 2 out]
          n408 = Select(t=w1084, s=w1085, f=cluster{dbl[], dbl[]} {[], []} ("s? t:f")) -> (s? t:f=w1077:cluster{dbl[], dbl[]})
          n409 = Build Array(w1088, w1077) -> (→"Detektor 2":cluster{dbl[], "ECD2Chrom":dbl[]}[])
        }
        n410 = global read "GVZeitenZyklen.vi" "Big Ben, Methodenzeit, Zykluszeit0, Zykluszeit1, Zykluszeit2A, Zykluszeit2B"() -> (w949:dbl[])
        n411 = Index Array(array=w949, index=3 ("Index")) -> (element=w947:dbl)
        n412 = while {
          tunnel: w991 -> [w1018]
          tunnel: w990 -> [w1017]
          tunnel: w912 -> [w1032]
          shift-right: [w1033] -> w984
          shift-left: w989 -> [w1034]
          tunnel: w909 -> [w1028]
          tunnel: w908 -> [w1022]
          shift-right: [w1019] -> _
          shift-left: w947 -> [w1023]
          stop <- w1035 stop-if-true
          n413 = Less?(x=w1023, y=w1028) -> (x < y?=w1026:bool)
          n414 = Less?(x=w1023, y=w1022) -> (x < y?=w1024:bool)
          n415 = call "Bis zum nächsten Vielfachen warten13"("Count(mSec)"=u32 100 ("Zu wartende ms")) -> ()  [unwired: 1 out]
          n416 = global read "GVMethodenwechsel.vi" "Methodenwechsel?"() -> (w1037:bool)
          n417 = global read "gvbooleschRT.vi" "global stop RT"() -> (w1038:bool)
          n418 = local read "veränderte Methode benutzen"() -> (w1036:bool)
          n419 = global read "GVZeitenZyklen.vi" "Big Ben, Methodenzeit, Zykluszeit0, Zykluszeit1, Zykluszeit2A, Zykluszeit2B"() -> (w1030:dbl[])
          n420 = Compound Arithmetic op=OR(w1038, w1037, w1036) -> (w1035:bool)
          n421 = Index Array(array=w1030, index=3 ("Index")) -> (element=w1019:dbl)
          n422 = Greater Or Equal?(x=w1019, y=w1028) -> (x >= y?=w1027:bool)
          n423 = Greater Or Equal?(x=w1019, y=w1022) -> (x >= y?=w1025:bool)
          n424 = And(x=w1025, y=w1024) -> (x .and. y?=w1021:bool)
          n425 = And(x=w1027, y=w1026) -> (x .and. y?=w1016:bool)
          n426 = Or(x=w1016, y=w1021) -> (x .or. y?=w1020:bool)
          n427 = And(x=w1032, y=w1020) -> (x .and. y?=w1031:bool)
          n428 = case shown="True" w1031 {
            tunnel: w1034 -> [w1040 w1041]
            tunnel: [w1040 w1045] -> w1033
            tunnel: w1018 -> [_ w1044]
            tunnel: w1017 -> [_ w1043]
            tunnel: w1016 -> [_ w1042]
            frame False {
            }
            frame True {
              n429 = call "MSDateienSchicken12-15.vi"("MSNummer"=w1041, "MSa?"=w1042, "Dateipfad:fromcriordy"=w1043, "Dateipfad:fromcriocmd"=w1044) -> ()  [unwired: 1 in]
              n430 = Increment(x=w1041) -> (x+1=w1045:i32)
            }
          }
        }
      }
      n431 = Add Array Elements(numeric array=w463) -> (sum=w473:i32)
      n432 = Index Array(array=w463, index #1=0 ("Index"), index #2=1 ("Index")) -> (element #1=w484:i32, element #2=w482:i32)
      n433 = Split 1D Array(array=w462, index=w484) -> (first subarray=w488:dbl[], second subarray=w492:dbl[])
      n434 = Split 1D Array(array=w460, index=w484) -> (first subarray=w491:string[], second subarray=w493:string[])
      n435 = Split 1D Array(array=w461, index=w484) -> (first subarray=w481:string[], second subarray=w483:string[])
      n436 = Initialize Array(-1.0 ("Element"), w473) -> (w458:dbl[])
      n437 = Split 1D Array(array=w493, index=w482) -> (first subarray=w490:string[], second subarray=w489:string[])
      n438 = Split 1D Array(array=w492, index=w482) -> (first subarray=w487:dbl[], second subarray=w486:dbl[])
      n439 = Split 1D Array(array=w483, index=w482) -> (first subarray=w480:string[], second subarray=w479:string[])
      n440 = Bundle(w491, w490, w489, w488, w487, w486) -> (w485:T23)  [unwired: 1 in]
      n441 = Bundle(w481, w480, w479) -> (w478:cluster{string[], string[], string[]})  [unwired: 1 in]
      n442 = Initialize Array(0.0, 8 ("Dimension")) -> (w408:dbl[])
      n443 = Bundle(w477, w477, w477) -> (w476:cluster{i32, i32, i32})  [unwired: 1 in]
      n444 = Initialize Array("x", 8 ("Dimension")) -> (w413:string[])
      n445 = case shown="True" TRUE ("SerielleKomm.") {
        tunnel: bool[] [TRUE, TRUE, TRUE, TRUE, TRUE, TRUE, TRUE, TRUE] -> [_ w551]
        tunnel: w413 -> [_ w550]
        tunnel: w485 -> [_ w549]
        tunnel: w484 -> [_ w548]
        tunnel: w482 -> [_ w547]
        tunnel: w478 -> [_ w546]
        tunnel: w476 -> [_ w545]
        tunnel: w475 -> [_ w544]
        tunnel: w462 -> [_ w543]
        tunnel: w459 -> [_ w542]
        tunnel: w458 -> [_ w541]
        tunnel: w457 -> [_ w538]
        tunnel: w436 -> [_ w540]
        tunnel: w408 -> [_ w539]
        tunnel: w407 -> [_ w537]
        frame False {
        }
        frame True {
          n446 = while {
            tunnel: w538 -> [w562]
            tunnel: w537 -> [w555]
            shift-right: [w554] -> _
            shift-left: errorcluster {"status"=FALSE, "code"=0, "source"=""} ("error out") -> [w553]
            stop <- w564 stop-if-true
            n447 = String To Byte Array(string=w555) -> (unsigned byte array=w558:u8[])
            n448 = call "Warten6"("Count(mSec)"=u32 500) -> ()  [unwired: 1 out]
            n449 = Join Numbers(hi=w558, lo=u8 5) -> ((hi.lo)=w560:u16[])
            n450 = Join Numbers(hi=w558, lo=u8 6) -> ((hi.lo)=w556:u16[])
            n451 = xnode "Invoke Method"("FPGA VI Reference In"=w562, "error in"=w553, "Data"=w560) -> ("FPGA VI Reference Out"=w559:refnum<k20>, "error out"=w552:errorcluster)  [unwired: 1 in, 1 out]
            n452 = xnode "Invoke Method"("FPGA VI Reference In"=w559, "error in"=w552, "Data"=w556) -> ("error out"=w554:errorcluster)  [unwired: 1 in, 2 out]
            "FIFOwriteRS485" <- w554
            n453 = global read "gvbooleschRT.vi" "global stop RT"() -> (w564:bool)
          }
          n454 = while {
            shift-right: [w702] -> _
            shift-left: w551 -> [w717]
            shift-right: [w721] -> _
            shift-left: w541 -> [w727]
            tunnel: w538 -> [w716]
            shift-right: [w703] -> _
            shift-left: w550 -> [w705]
            tunnel: w542 -> [w707]
            tunnel: w543 -> [w704]
            shift-right: [w708] -> _
            shift-left: w544 -> [w723]
            tunnel: w548 -> [w725]
            tunnel: w547 -> [w726]
            tunnel: w549 -> [w728]
            tunnel: w546 -> [w710]
            shift-right: [w709] -> _
            shift-left: w545 -> [w711]
            shift-right: [w714] -> _
            shift-left: w540 -> [w715]
            shift-right: [w718] -> _
            shift-left: w539 -> [w719]
            shift-right: [w699] -> _
            shift-left: errorcluster {"status"=FALSE, "code"=0, "source"=""} ("error out") -> [w698]
            stop <- w722 stop-if-true
            n455 = for {
              tunnel: w717 -> [w732] mode=indexing
              tunnel: w719 -> [w729] mode=indexing
              tunnel: [w736] -> w718 mode=indexing
              tunnel: [w733] -> w712 mode=indexing
              n456 = global read "GVZeitenZyklen.vi" "Big Ben, Methodenzeit, Zykluszeit0, Zykluszeit1, Zykluszeit2A, Zykluszeit2B"() -> (w739:dbl[])
              n457 = Index Array(array=w739, index=0 ("Index")) -> (element=w737:dbl)
              n458 = Subtract(x=w737, y=w729) -> (x-y=w735:dbl)
              n459 = Greater?(x=w735, y=0.1) -> (0:w731:bool)
              n460 = Or(x=w732, y=w731) -> (x .or. y?=w730:bool)
              n461 = Select(t=w731, s=w731, f=w732) -> (s? t:f=w733:bool)
              n462 = Select(t=w737, s=w730, f=w729) -> (s? t:f=w736:dbl)
            }
            n463 = global read "GVHorstSP.vi" "HorstSP"() -> (w721:dbl[])
            n464 = Not Equal?(x=w721, y=w727) -> (x != y?=w724:bool)
            n465 = call "NeueSP.vi"("Anzahl2"=w726, "Anzahl1"=w725, "AlteSP"=w727, 7:"NeueSP"=w721, "BefehleCluster"=w723, 10:"NeueSP"=w724, "ClusterFest"=w728) -> ("BefehleCluster"=w713:T24)  [unwired: 4 in]
            n466 = call "Warten3"("Count(mSec)"=u32 50) -> ()  [unwired: 1 out]
            n467 = call "MPVSenden-01-17.vi"("Ventilposition"=w715, "error in"=w698, "FPGA VI Reference In"=w716) -> ("Ventilposition"=w714:i32, "error out"=w701:errorcluster, "FPGA VI Reference Out"=w697:refnum<k20>)
            n468 = call "Senden-01-17.vi"("error in"=w701, "BefehlsCluster"=w713, "AbfragenCluster"=w710, "Abfragenr.Cluster"=w711, "Senden?"=w712, "FPGA VI Reference In"=w697) -> ("BefehlsCluster"=w708:T24, "error out"=w700:errorcluster, "Senden?"=w706:bool[], "Abfragenr.Cluster"=w709:cluster{i32, i32, i32})  [unwired: 1 in]
            n469 = call "SeriellRead-01-17.vi"("SkalierungsfaktorHorst"=w704, "VorwortHorst"=w707, "error in"=w700, "Zwischenspeicher"=w705, "Senden?"=w706, "FPGA VI Reference In"=w697) -> ("Senden?"=w702:bool[], "Zwischenspeicher"=w703:string[], "error out"=w699:errorcluster)  [unwired: 3 in]
            "SerielleKomm." <- w699
            n470 = global read "gvbooleschRT.vi" "global stop RT"() -> (w722:bool)
          }
        }
      }
    }
    frame #2 {
      n471 = xnode "Read/Write Control"("FPGA VI Reference In"=w1270, "global stop"=TRUE) -> ("FPGA VI Reference Out"=w1269:refnum<k20>)  [unwired: 1 in, 1 out]
      n472 = xnode "Close FPGA VI Reference"("FPGA VI Reference In"=w1269) -> ()  [unwired: 1 in, 1 out]
    }
  }
